vi "LabVIEW-Int_Buck_Boost_Inverter_PI_v0.3.2_9Aug2020.vi"() -> ()   [LabVIEW 2018]
uses:
  <vilib>/Modbus/master/Create Master Instance (TCP).vi
  <vilib>/Modbus/master/Create Master Instance (Serial).vi
  <vilib>/Modbus/master/Modbus Master.lvclass
panel:
  out "Future_5":sgl=1257163500000.0
  out "Future_6":sgl=-2.1506243e+28
  out "Future_4":sgl=84.72166
  out "Future_2":sgl=1.1313919e+38
  out "Future_3":sgl=5.1706567e-10
  out "RMS_V_CA":sgl=1.8692774
  out "Future_1":sgl=3.3164534e-12
  out "RMS_V_BC":sgl=1.8672488
  out "Avg_F_Grid":sgl=60.10614
  out "RMS_V_AB":sgl=1.5779244
  out "Avg_V_Boost":sgl=23.65672
  out "Avg_I_Boost":sgl=-0.037957944
  out "Avg_I_Buck":sgl=0.064867415
  out "Avg_I_DC_In":sgl=0.2081415
  out "Avg_V_Buck":sgl=0.6698118
  out "spll1.theta":sgl=0.025031969
  out "Avg_V_DC_In":sgl=23.77852
  out "Step_sin":sgl=2.9028316
  out "Sine2":sgl=45.3112
  out "Sine3":sgl=1937.8336
  out "V_CA":sgl=0.9757843
  out "Sine1":sgl=1390.5049
  out "V_BC":sgl=-0.4336853
  out "SPI-ADC2_V7":sgl
  out "V_AB":sgl=-0.542099
  out "SPI-ADC2_V5":sgl
  out "SPI-ADC2_V6":sgl
  out "SPI-ADC2_V4":sgl
  out "SPI-ADC2_V2":sgl
  out "SPI-ADC2_V3":sgl
  out "SPI-ADC2_V0":sgl
  out "SPI-ADC2_V1":sgl
  out "SPI-ADC1_V6":sgl
  out "SPI-ADC1_V7":sgl
  out "SPI-ADC1_V5":sgl
  out "SPI-ADC1_V3":sgl
  out "SPI-ADC1_V4":sgl
  out "SPI-ADC1_V1":sgl
  out "SPI-ADC1_V2":sgl
  out "SPI-ADC1_V0":sgl
  out "Ia":sgl=0.07590008
  out "I_L5":sgl=0.009900093
  out "I_Buck":sgl=0.0692997
  out "I_Boost":sgl=-0.0033006668
  out "I_L3":sgl=0.029699326
  out "I_L1":sgl=0.0692997
  out "I_L2":sgl=0.082499504
  out "ADCB7":sgl
  out "I_DCin2":sgl=-0.06270027
  out "ADCB6":sgl
  out "ADCB4":sgl
  out "ADCB5":sgl
  out "ADCB2":sgl
  out "ADCB3":sgl
  out "V_DCin":sgl=23.53728
  out "V_PhA":sgl=-0.7824631
  out "V_PhC":sgl=1.114891
  out "V_PhB":sgl=-1.1619263
  out "V_Buck":sgl=0.64584
  out "I_DCin":sgl=0.23429966
  out "V_Boost":sgl=23.322
  out "ADCB0":sgl
  out "V_Pot":sgl=0.030416729
  out "ADCB1":sgl
  out "Status_Registers":u16[](array[numeric])
  out "DL_RegValues":u16[](array[numeric])=[49325, 30936, 49424, 55648, 49396, 39032, 49437, 56332, 49509, 55732, 49416, 11504, 49415, 20192, 49485, 36984, 49430, 3488, 49418, 50960, 49456, 61696, 49523, 47720, 49458, 44316, 49377, 33664, 49468, 14228, 49465, 40308, 49398, 21648, 49417, 59656, 49479, 32296, 49482, 6216, 49496, 55056, 49468, 14228, 49510, 47040, 49454, 22240, 49490, 50364, 49453, 30928, 49430, 60336, 49430, 60336, 49438, 47632, 49410, 6816, 49440, 30256, 49289, 2800]
  out "Array":sgl[](array[numeric])=[1678.6465, 1616.1086, 1551.6309, 1485.4673, 1417.8794, 1349.1339, 1279.5023, 1209.259, 1138.6813, 1068.048, 997.6377, 927.7282, 858.59503, 790.512, 723.7472, 658.5642, 595.22015, 533.9653, 475.041, 418.67975, 365.1046, 314.5266, 267.1455, 223.14833, 182.70808, 145.98491, 113.12389, 84.2547, 59.490856, 38.93016, 22.654057, 10.726688, 3.1949756, 0.08881263, 1.4203317, 7.184372, 17.358076, 31.901361, 50.756786, 73.85028, 101.09016, 132.36922, 167.56369, 206.53542, 249.12988, 295.1792, 344.50198, 396.90262, 452.1756, 510.1018, 570.45294, 632.99084, 697.4691, 763.6325, 831.2203, 899.96564, 969.59735, 1039.8402, 1110.4181, 1152.81, 1223.3429, 1293.4861, 1362.9624, 1431.4979, 1498.822, 1564.6691, 1628.7792, 1690.8993, 1750.7843, 1808.1979, 1862.9133, 1914.7147, 1963.398, 2008.7705, 2050.6533, 2088.8813, 2123.3037, 2153.7842, 2180.203, 2202.4556, 2220.454, 2234.1277, 2243.422, 2248.3008, 2248.7446, 2244.752, 2236.3381, 2223.5369, 2206.3982, 2184.99, 2159.3965, 2129.7195, 2096.075, 2058.5967, 2017.432, 1972.7434, 1924.7074, 1873.5137, 1819.3641, 1762.4723, 1703.0629, 1641.3706, 1577.6385, 1512.1184, 1445.0685, 1376.7539, 1307.4437, 1237.412, 1166.9349, 1096.2902, 1025.7573, 955.61383, 886.1375, 817.6021, 750.27795, 684.431, 620.32104, 558.2009, 498.31558, 440.90207, 386.18668, 334.38516, 285.70212, 240.32965, 198.44649, 160.21844, 125.79642, 95.31566, 68.89695, 46.64446, 28.645927, 14.972402, 5.6778417, 0.79904556, 0.35511646, 4.3479314, 12.761537, 25.563023, 42.701714, 64.10992, 89.70303, 119.380196, 153.02469, 190.50308, 231.66771, 276.35614, 324.39224, 375.586, 429.73557, 486.62726, 546.0365, 607.7292, 671.4613, 736.9814, 804.0311, 872.3454, 941.6553, 1011.6875, 1082.1652, 1124.5499, 1195.161, 1265.4934, 1335.2695, 1404.2141, 1472.0549, 1538.5243, 1603.3599, 1666.306, 1727.1139, 1785.5438, 1841.365, 1894.3573, 1944.3115, 1991.0305, 2034.3298, 2074.0388, 2110.0005, 2142.0732, 2170.13, 2194.0603, 2213.77, 2229.181, 2240.2324, 2246.8806, 2249.0999, 2246.8809, 2240.2324, 2229.181, 2213.77, 2194.0603, 2170.1301, 2142.0732, 11.81778, 11.655151, 10.083061, 12.576717, 12.79356, 8.782017, 12.847767, 6.722042, 7.80624, 7.8604507, 8.294132, 5.9630966, 3.7947006, 5.7462616, 4.391014, 2.4394493, 1.4636726, -0.10841751, 2.331028, -3.5778618, -2.3852425, -2.7647057, -4.662056, -6.4509926, -5.6378365, -9.595173, -10.896214, -13.552502, -14.203022, -16.8051, -14.745121, -12.305668, -16.20879, -17.835094, -20.166122, -17.78088, -19.73244, -16.371422, -19.461388, -19.190342, -20.708221, -18.485611, -18.756657, -16.371418, -19.407177, -17.997715, -18.75666, -17.83509, -16.15458, -16.58826, -14.257233, -16.750885, -13.606712, -18.106136, -13.823547, -12.522507, -12.739349, -14.203026, -14.148811, -12.305664, -11.709358, -11.329895, -10.733582, -7.6978226, -7.643608, -10.028854, -9.703587, -8.40255, -5.0957413, -6.993088, -5.475212, -5.2583694, -6.234146, -2.276825, -0.2710495, 0.8131485, 2.5478668, 3.6862793, 5.3125763, 6.396782, 10.950417, 8.239922, 9.595169, 8.998863, 13.010403, 11.546734, 13.931969, 10.245693, 14.040386, 10.516739, 15.070381, 11.926201, 10.787788, 11.54673, 10.462528, 11.438309, 9.812008, 13.173031, 13.769337, 11.167263, 8.836227, 9.595173, 12.197254, 9.378334, 12.847771, 11.004627, 9.812012, 11.329891, 8.619392, 8.890438, 8.40255, 7.0472984, 8.998856, 4.824688, 3.4152298, 4.5536423, 4.1741676, 2.8189201, -3.198391, -1.3010406, -0.542099, -2.6020813, -1.409462, -6.55941, -8.023079, -7.752033, -12.739349, -13.877758, -11.81778, -13.44408, -15.449848, -13.498287, -15.93774, -19.35297, -17.45562, -19.08192, -19.136127, -19.298756, -20.057697, -21.955048, -20.437168, -19.786652, -18.377193, -16.750893, -15.612484, -16.859314, -21.467163, -16.750893, -16.47984, -17.40141, -15.124588, -14.8535385, -15.775108, -15.124592, -14.528282, -17.238777, -12.847771, -13.606712, -14.745121, -10.137268, -12.901978, -12.414085, -10.950417, -9.757797, -7.8062363, -13.227238, -8.077293, -6.3425674, -7.914665, -5.6378403, -3.361023, -4.7162704, -3.3610153, -1.8973465, 0.43367767, -0.05420685, -1.1384125, 1.3552475, 4.7704773, 7.8604507, 7.1015167, 9.32412, 10.408325, 8.456757, 13.660919, 11.655148, 13.660923, 12.305668, 14.961956, 11.275677, 14.203022, 12.685139, -15.341431, -13.11882, -13.38987, -16.100368, -14.961964, -15.178799, -15.341427, -17.889301, -15.829319, -15.341431, -19.949284, -17.292992, -17.076149, -18.702446, -16.046158, -16.913525, -15.28722, -15.558273, -18.810871, -13.7693405, -15.016167, -13.11882, -12.4683, -10.625153, -13.498291, -12.847763, -9.486748, -6.396782, -6.5051956, -3.4152298, -4.933113, -3.903122, -0.8131485, -0.7047272, 1.8431473, 2.7647095, 2.276825, 0.8131561, 3.8489075, 5.90889, 6.993088, 9.107285, 8.023079, 7.860443, 9.378326, 10.950417, 14.745125, 11.384102, 14.8535385, 12.305672, 11.438309, 13.823547, 14.582493, 15.666687, 13.931969, 17.13036, 16.696682, 20.870853, 20.057705, 19.895065, 16.85931, 19.895073, 19.786648, 19.515602, 18.322979, 17.618252, 15.504059, 16.15458, 17.50983, 14.36565, 15.829319, 13.552498, 14.203018, 12.847771, 12.576721, 10.679371, 8.890438, 10.841999, 6.938881, 7.0472946, 4.282593, 3.1441803, 1.8431435, 2.2226105, 1.1926193, -1.029995, 0.0, -0.704731, -5.854679, -5.7462616, -8.239922, -8.348343, -7.2099304, -8.782021, -10.841999, -9.757797, -6.5051994, -12.685139, -16.154583, -11.709362, -13.7693405, -11.980412, -11.655148, -14.8535385, -16.317207, -18.214558, -14.8535385, -14.582485, -18.919289, -18.4314, -14.257233, -16.913517, -19.29876, -17.021938, -16.85931, -18.214561, -17.835087, -18.648243, -13.606705, -13.335663, -14.203018, -10.516739, -14.04039, -15.124588, -12.630928, -6.938881, -7.155716, -4.824692, -9.649376, -7.8062363, -1.8431396, -9.757805, -2.7647095, -0.6505203, -2.3852386, -0.8131485, 3.9031143, 3.9031143, 3.7947006, 4.9331055, 8.239914, 8.673599, 8.348343, 5.8004684, 10.950424, 10.354111, 10.462532, 10.137268, 12.739349, 14.257233, 10.950417, 13.7693405, 15.991951, 14.365654, 16.642471, 18.594028, 17.13036, 16.371418, 19.94928, 17.50983, 18.322979, 21.467155, 18.594028, 19.62402, 22.171886, 21.738209, 16.53405, 19.190338, 17.292992, 14.3114395, 14.419861, 19.94928, 14.528278, 8.944649, 11.329891, 11.655148, 8.836235, 7.264145, 7.6978226, 4.7704773, 6.450989, 2.4394493, 4.0115356, 2.4394531, -0.48788834, -0.8131523, -4.228382, -2.873127, -5.0415306, -3.1441765, -4.1741676, -8.402554, 3.5236511, 1.4636688, 3.3068085, 3.5236511, 2.1684036, 6.396782, 2.49366, 11.167259, 8.023079, 7.48098, 11.655151, 11.329895, 13.281448, 12.956184, 11.655144, 14.474075, 13.823547, 15.666691, 16.479843, 17.347202, 17.40141, 15.883526, 17.130356, 17.076145, 19.136127, 22.442936, 20.382961, 19.949284, 20.708218, 20.22033, 19.678234, 16.20879, 17.021938, 18.539822, 18.322975, 15.0161705, 17.455616, 15.558266, 15.61248, 13.281452, 13.715134, 9.378326, 10.733578, 8.510975, 10.028851, 7.0472984, 4.0115356, 6.450989, 1.3010406, 4.282589, 2.818924, 2.9273376, -0.9757805, 2.4394493, -0.108421326, -4.607853, -3.9573326, -6.6678276, -5.9088936, -7.5894012, -5.149952, -8.565178, -9.053066, -11.81778, -10.679371, -7.5893974, -5.8004723, -7.7520294, -12.414089, -7.3725624, -10.354107, -8.294128, -7.968872, -10.570946, -12.305672, -11.492519, -11.438305, -14.528278, -12.251457, -13.444077, -15.233009, -11.384102, -11.438313, -11.221474, -14.203022, -10.516739, -13.931969, -9.540962, -8.185707, -4.7704773, -6.8304596, -3.577858, -3.577858, -2.7647095, 0.37947083, -1.6805115, -3.3068085, -0.48789215, 2.3852463, 0.542099, 4.933113, 2.3852386, -0.5421066, 5.4752045, 3.4694366, 7.2099304, 5.041527, 3.252594, 10.299896, 9.540962, 5.854683, 9.866219, 10.299904, 12.19725, 13.44408, 13.660919, 13.660919, 15.829323, 16.805096, 14.6367035, 14.745117, 13.11882, 15.449852, 21.683998, 20.654007, 14.690914, 19.895065, 18.70245, 21.467155, 21.250317, 17.292988, 23.256092, 18.70245, 20.00349, 19.840858, 19.89507, 15.233013, 15.395641, 16.262997, 17.021942, 12.197254, 11.113052, 10.028851, 10.950424, 4.66206, 6.5052032, 11.004631, 6.6136246, 3.74049, 3.1441765, 4.1741714, 1.084198, -0.21684265, 0.75893784, -2.1141891, -1.3552513, -4.282589, -2.7647057, -5.204159, -7.3725624, -5.4210014, -9.05307, -7.643612, -9.866222, -14.36565, -8.510971, -8.456757, -12.847771, -9.378326, -8.673599, -11.058838, -15.233009, -11.167263, -7.0473022, -11.763569, -11.600941, -7.6978226, -8.619392, -12.4683, -12.630928, -13.5525055, -11.763569, -14.419861, -10.89621, -13.173031, -10.841995, -9.432541, -9.432541, -9.920425, -8.1315, -10.028854, -4.282585]
  out "output array":u16[](array[numeric])=[17617, 54448, 17610, 890, 17601, 62512, 17593, 44788, 17585, 15396, 17576, 42057, 17567, 61459, 17559, 10314, 17550, 21965, 17541, 33161, 17529, 26832, 17511, 61083, 17494, 42517, 17477, 41157, 17460, 61394, 17444, 42012, 17428, 52759, 17413, 32199, 17389, 34111, 17361, 22274, 17334, 36196, 17309, 17256, 17285, 37536, 17247, 9721, 17206, 46405, 17169, 64547, 17122, 16239, 17064, 33384, 17005, 63139, 16923, 47228, 16821, 15234, 16683, 41092, 16460, 31355, 15797, 58213, 16309, 52590, 16613, 58976, 16778, 56663, 16895, 13821, 16971, 1779, 17043, 45912, 17098, 11817, 17156, 24197, 17191, 36942, 17230, 35089, 17273, 8512, 17299, 38640, 17324, 16449, 17350, 29577, 17378, 5754, 17407, 3336, 17422, 40189, 17438, 16234, 17454, 24070, 17470, 59515, 17487, 52761, 17504, 64973, 17522, 26171, 17537, 64227, 17546, 52577, 17552, 6636, 17560, 60153, 17569, 44942, 17578, 24268, 17586, 61423, 17595, 23118, 17603, 38249, 17611, 39151, 17619, 23751, 17626, 55577, 17634, 1621, 17640, 56634, 17647, 22239, 17653, 27836, 17659, 6312, 17664, 10868, 17666, 36378, 17668, 46300, 17670, 40076, 17672, 17215, 17673, 42826, 17674, 51012, 17675, 41483, 17676, 14017, 17676, 34000, 17676, 35818, 17676, 19464, 17675, 50537, 17674, 63639, 17673, 58975, 17672, 36823, 17670, 63064, 17669, 7043, 17667, 307, 17664, 43404, 17660, 11731, 17654, 38858, 17648, 38563, 17642, 12400, 17635, 27559, 17628, 20253, 17620, 57859, 17613, 11228, 17605, 13423, 17597, 970, 17588, 41521, 17580, 6176, 17571, 28211, 17562, 44335, 17553, 56811, 17545, 2377, 17536, 14396, 17518, 59209, 17501, 35021, 17484, 26249, 17467, 37322, 17451, 7062, 17435, 5260, 17419, 36060, 17401, 10341, 17372, 29559, 17345, 6117, 17319, 12621, 17294, 55775, 17264, 21604, 17222, 29261, 17184, 14316, 17147, 38852, 17086, 41374, 17033, 52029, 16954, 37869, 16869, 10972, 16751, 36597, 16565, 45281, 16204, 36416, 16053, 53715, 16523, 8769, 16716, 12097, 16844, 33042, 16938, 52878, 17024, 14407, 17075, 26612, 17134, 49833, 17177, 1618, 17214, 32970, 17255, 43759, 17290, 11670, 17314, 12853, 17339, 51970, 17366, 56871, 17395, 20554, 17416, 33366, 17431, 61099, 17447, 56710, 17464, 16079, 17481, 510, 17498, 5659, 17515, 27120, 17532, 60416, 17543, 17737, 17548, 37273, 17557, 25895, 17566, 12234, 17574, 59552, 17583, 34522, 17592, 450, 17600, 20679, 17608, 27524, 17616, 18891, 17623, 58277, 17631, 12647, 17638, 11182, 17644, 52079, 17651, 2552, 17656, 57594, 17662, 19086, 17665, 41119, 17667, 57346, 17669, 57644, 17671, 41492, 17673, 8439, 17674, 23634, 17675, 21221, 17676, 952, 17676, 28183, 17676, 37273, 17676, 28184, 17676, 952, 17675, 21221, 17674, 23634, 17673, 8439, 17671, 41493, 17669, 57644, 16701, 5536, 16698, 31616, 16673, 21560, 16713, 14908, 16716, 45676, 16652, 33572, 16717, 36980, 16599, 6904, 16633, 52408, 16635, 35024, 16644, 46276, 16574, 53680, 16498, 56416, 16567, 57696, 16524, 33584, 16412, 8176, 16315, 22944, 48606, 2560, 16405, 12176, 49252, 64432, 49176, 42960, 49200, 61680, 49301, 12176, 49358, 28296, 49332, 26920, 49433, 34260, 49454, 22244, 49496, 55052, 49507, 16276, 49542, 28888, 49515, 60420, 49476, 58372, 49537, 43930, 49550, 44614, 49569, 21560, 49550, 16190, 49565, 56330, 49538, 63660, 49563, 45292, 49561, 34258, 49573, 43632, 49555, 57992, 49558, 3490, 49538, 63658, 49563, 16870, 49551, 64338, 49558, 3492, 49550, 44612, 49537, 15508, 49540, 46274, 49508, 7584, 49542, 464, 49497, 46360, 49552, 55646, 49501, 11584, 49480, 23600, 49483, 54368, 49507, 16280, 49506, 24968, 49476, 58368, 49467, 22920, 49461, 18240, 49451, 48320, 49398, 21648, 49396, 39024, 49440, 30256, 49435, 16868, 49414, 28888, 49315, 4176, 49375, 51040, 49327, 13552, 49320, 17552, 49351, 32288, 49169, 46976, 48778, 50944, 16208, 10880, 16419, 4160, 16491, 60416, 16554, 160, 16588, 45680, 16687, 13544, 16643, 54968, 16665, 34256, 16655, 64344, 16720, 10908, 16696, 49004, 16734, 59736, 16675, 61020, 16736, 42348, 16680, 17552, 16753, 8264, 16702, 53688, 16684, 39624, 16696, 49000, 16679, 26244, 16695, 848, 16668, 65020, 16722, 50364, 16732, 20276, 16690, 44316, 16653, 24880, 16665, 34260, 16707, 10228, 16662, 3496, 16717, 36984, 16688, 4852, 16668, 65024, 16693, 18236, 16649, 59656, 16654, 16188, 16646, 28888, 16609, 33656, 16655, 64336, 16538, 25560, 16474, 37664, 16529, 46960, 16517, 37576, 16436, 26928, 49228, 45680, 49062, 34944, 48906, 50944, 49190, 34944, 49076, 26944, 49361, 59056, 49408, 24200, 49400, 4264, 49483, 54368, 49502, 2892, 49469, 5536, 49495, 6900, 49527, 12948, 49495, 63740, 49535, 252, 49562, 53986, 49547, 42268, 49560, 42950, 49561, 5834, 49562, 25562, 49568, 30250, 49583, 41968, 49571, 32594, 49566, 19216, 49555, 1150, 49542, 468, 49529, 52412, 49542, 57312, 49579, 48320, 49542, 468, 49539, 54966, 49547, 13846, 49521, 65104, 49517, 43032, 49532, 26328, 49521, 65108, 49512, 29656, 49545, 59652, 49485, 36984, 49497, 46360, 49515, 60420, 49442, 12864, 49486, 28288, 49478, 40984, 49455, 13544, 49436, 8176, 49401, 52400, 49491, 41668, 49409, 15512, 49354, 63056, 49405, 17648, 49332, 26928, 49239, 6912, 49302, 60336, 49239, 6880, 49138, 56384, 16094, 2816, 48478, 2048, 49041, 46976, 16301, 30912, 16536, 42944, 16635, 35024, 16611, 16288, 16661, 12184, 16678, 34944, 16647, 20192, 16730, 37664, 16698, 31612, 16730, 37668, 16708, 58372, 16751, 25644, 16692, 26924, 16739, 16276, 16714, 63060, 49525, 30336, 49489, 59056, 49494, 15592, 49536, 52622, 49519, 25652, 49522, 56412, 49525, 30332, 49551, 7498, 49533, 17636, 49525, 30336, 49567, 38946, 49546, 22540, 49544, 39924, 49557, 40604, 49536, 24200, 49543, 20198, 49524, 39028, 49528, 61104, 49558, 31914, 49500, 20280, 49520, 16952, 49489, 59056, 49479, 32296, 49450, 160, 49495, 63744, 49485, 36976, 49431, 51640, 49356, 45680, 49360, 10896, 49242, 37664, 49309, 56336, 49273, 52416, 48976, 10880, 48948, 26880, 16363, 60480, 16432, 61696, 16401, 46976, 16208, 11008, 16502, 21632, 16573, 5536, 16607, 51040, 16657, 46960, 16640, 24200, 16635, 35008, 16662, 3488, 16687, 13544, 16747, 60424, 16694, 9544, 16749, 43032, 16708, 58376, 16695, 848, 16733, 11584, 16745, 20964, 16762, 43712, 16734, 59736, 16777, 2810, 16773, 37582, 16806, 63362, 16800, 30254, 16799, 10520, 16774, 57310, 16799, 10524, 16798, 19214, 16796, 8180, 16786, 38262, 16780, 61998, 16760, 4256, 16769, 15508, 16780, 5154, 16741, 55732, 16765, 17636, 16728, 55048, 16739, 16272, 16717, 36984, 16713, 14912, 16682, 57012, 16654, 16188, 16685, 30932, 16606, 2896, 16609, 33648, 16521, 2816, 16457, 14912, 16363, 60448, 16398, 16192, 16280, 42944, 49027, 55008, 0, 0, 48948, 26944, 49339, 22920, 49335, 57696, 49411, 54968, 49413, 37584, 49382, 47040, 49420, 33576, 49453, 30932, 49436, 8176, 49360, 10904, 49482, 63060, 49537, 15510, 49467, 22924, 49500, 20280, 49471, 44996, 49466, 31612, 49517, 43032, 49538, 35236, 49553, 46954, 49517, 43032, 49513, 20956, 49559, 23220, 49555, 29570, 49508, 7584, 49543, 20194, 49562, 25564, 49544, 11502, 49542, 57310, 49553, 46956, 49550, 44610, 49557, 12186, 49497, 46352, 49493, 24288, 49507, 16272, 49448, 17552, 49504, 42352, 49521, 65104, 49482, 6216, 49374, 2896, 49380, 64416, 49306, 25568, 49434, 25560, 49401, 52400, 49131, 60416, 49436, 8184, 49200, 61696, 48934, 34944, 49176, 42944, 48976, 10880, 16505, 52384, 16505, 52384, 16498, 56416, 16541, 56320, 16643, 54960, 16650, 50960, 16645, 37584, 16569, 40304, 16687, 13552, 16677, 43632, 16679, 26248, 16674, 12864, 16715, 54368, 16740, 7584, 16687, 13544, 16732, 20280, 16767, 57096, 16741, 55736, 16773, 9160, 16788, 49298, 16777, 2810, 16770, 63658, 16799, 38944, 16780, 5154, 16786, 38262, 16811, 48316, 16788, 49298, 16796, 65022, 16817, 24582, 16813, 59354, 16772, 17852, 16793, 34256, 16778, 22540, 16740, 64424, 16742, 47040, 16799, 38944, 16744, 29652, 16655, 7496, 16693, 18236, 16698, 31612, 16653, 24888, 16616, 29664, 16630, 21648, 16536, 42944, 16590, 28288, 16412, 8176, 16512, 24192, 16412, 8192, 48889, 52352, 48976, 10944, 49287, 20200, 49207, 57680, 49313, 21560, 49225, 14896, 49285, 37576, 49414, 28892, 16481, 33664, 16315, 22912, 16467, 41664, 16481, 33664, 16394, 50976, 16588, 45680, 16415, 38944, 16690, 44312, 16640, 24200, 16623, 25648, 16698, 31616, 16693, 18240, 16724, 32976, 16719, 19592, 16698, 31608, 16743, 38352, 16733, 11584, 16762, 43716, 16771, 54968, 16778, 50962, 16779, 13846, 16766, 8940, 16777, 2808, 16776, 39922, 16793, 5834, 16819, 35618, 16803, 4174, 16799, 38946, 16805, 43630, 16801, 49980, 16797, 27910, 16769, 43930, 16776, 11502, 16788, 20878, 16786, 38260, 16752, 16956, 16779, 42266, 16760, 61096, 16761, 52408, 16724, 32980, 16731, 28976, 16662, 3488, 16683, 48316, 16648, 11508, 16672, 30252, 16609, 33656, 16512, 24192, 16590, 28288, 16294, 34944, 16521, 2808, 16436, 26944, 16443, 22912, 49017, 52416, 16412, 8176, 48606, 3072, 49299, 29576, 49277, 17648, 49365, 24280, 49341, 5544, 49394, 56416, 49316, 52328, 49417, 2808, 49424, 55644, 49469, 5536, 49450, 57012, 49394, 56408, 49337, 40312, 49400, 4256, 49478, 40988, 49387, 60424, 49445, 43628, 49412, 46272, 49407, 256, 49449, 8856, 49476, 58376, 49463, 57692, 49463, 844, 49512, 29652, 49476, 1528, 49495, 6896, 49523, 47720, 49462, 9544, 49463, 852, 49459, 35624, 49507, 16276, 49448, 17552, 49502, 59736, 49432, 42952, 49410, 63656, 49304, 42944, 49370, 37664, 49252, 64416, 49252, 64416, 49200, 61696, 16066, 18944, 49111, 6912, 49235, 41664, 48889, 52480, 16408, 42976, 16138, 50944, 16541, 56336, 16408, 42944, 48906, 51072, 16559, 13536, 16478, 2880, 16614, 47040, 16545, 21552, 16464, 10880, 16676, 52320, 16664, 42952, 16571, 22928, 16669, 56328, 16676, 52328, 16707, 10224, 16727, 6900, 16730, 37664, 16730, 37664, 16765, 17640, 16774, 28886, 16746, 12272, 16747, 60416, 16721, 59056, 16759, 12952, 16813, 30932, 16805, 15208, 16747, 3580, 16799, 10520, 16789, 40606, 16811, 48316, 16810, 166, 16778, 22538, 16826, 3194, 16789, 40606, 16800, 1830, 16798, 47636, 16799, 10522, 16755, 47724, 16758, 21644, 16770, 6814, 16776, 11504, 16707, 10228, 16689, 53008, 16672, 30252, 16687, 13552, 16533, 12184, 16592, 10912, 16688, 4856, 16595, 41680, 16495, 25648, 16457, 14896, 16517, 37584, 16266, 50944, 48734, 3072, 16194, 18880, 49159, 20192, 49069, 30944, 49289, 2808, 49200, 61680, 49318, 34936, 49387, 60424, 49325, 30936, 49424, 55648, 49396, 39032, 49437, 56332, 49509, 55732, 49416, 11504, 49415, 20192, 49485, 36984, 49430, 3488, 49418, 50960, 49456, 61696, 49523, 47720, 49458, 44316, 49377, 33664, 49468, 14228, 49465, 40308, 49398, 21648, 49417, 59656, 49479, 32296, 49482, 6216, 49496, 55056, 49468, 14228, 49510, 47040, 49454, 22240, 49490, 50364, 49453, 30928, 49430, 60336, 49430, 60336, 49438, 47632, 49410, 6816, 49440, 30256, 49289, 2800]
  in  "ARA-SGPN Interface Demo":enum32{"Control", "Datalogger"}(tab)
  in  "parity (None)":u16(ring) items=["None", "Odd", "Even"]
  in  "baud rate (115200)":u32=115200
  in  "unit ID":u8=1
  in  "serial type":enum16{"RTU", "ASCII"}(ring)
  in  "Serail Comm Port":refnum<visa-resource-name>="COM13"
  out "RX/TX_Errors":i16=52
  out "Modbus_Master-Error":errorcluster
  in  "IP Address":string="192.168.0.64"
  in  "CtrlSrc_Serial/nTCP":bool=TRUE
  in  "Inverter_Op-Mode":u16(ring)=1 items=["Passive", "Islanded", "Grid-Forming", "Grid-Feeding", "Grid-Supporting"]
  in  "AC Mag Ref (V)":fxp<+,16,11>=30.0
  in  "PWM_En":bool
  in  "PLL_Ki":fxp<+,16,6>=0.009765625
  in  "AC Power Ref (Q)":fxp<+,16,6>
  in  "PLL_Kp":fxp<+,16,6>=1.0
  in  "AC Freq Ref (Hz)":fxp<+,16,11>=60.0
  in  "AC Power Ref (P)":fxp<+,16,6>
  in  "Inv_Sw_Freq (kHz)":fxp<+,16,11>=30.0
  in  "Inv_En":bool
  in  "Buck_En":bool
  in  "Boost_En":bool
  in  "Buck_Op-Mode":u16(ring)=1 items=["Passive", "Voltage-Mode", "Current-Mode", "Dual-Loop"]
  in  "Buck_V_Ref (V)":fxp<+,16,6>=15.0
  in  "Buck_I_Kp":fxp<+,16,6>=1.0
  in  "Buck_V_Ki":fxp<+,16,6>=0.03125
  in  "Buck_I_Ki":fxp<+,16,6>=0.009765625
  in  "Buck_I_Ref (A)":fxp<+,16,6>
  in  "Buck_V_Kp":fxp<+,16,6>=1.0
  in  "Buck_Sw_Freq (kHz)":fxp<+,16,11>=30.0
  in  "Boost_Op-Mode":u16(ring)=1 items=["Passive", "Voltage-Mode", "Current-Mode", "Dual-Loop"]
  in  "Boost_V_Ref (V)":fxp<+,16,6>=36.0
  in  "Boost_I_Ki":fxp<+,16,6>=0.009765625
  in  "Boost_V_Ki":fxp<+,16,6>=0.03125
  in  "Boost_I_Ref (A)":fxp<+,16,6>
  in  "Boost_V_Kp":fxp<+,16,6>=1.0
  in  "Boost_Sw_Freq (kHz)":fxp<+,16,11>=30.0
  in  "Boost_I_Kp":fxp<+,16,6>=1.0
  out "V_Buck_FP":sgl=0.64584
  out "V_Boost_FP":sgl=23.322
  out "I_Boost_FP":sgl=-0.0033006668
  out "I_Buck_FP":sgl=0.0692997
  out "V_DCin_FP":sgl=23.53728
  out "I_DCin_FP":sgl=0.23429966
  out "V_Pot_FP":sgl=0.030416729
  out "RMS_V_AB_FP":sgl=1.5779244
  out "Avg_F_Grid_FP":sgl=60.10614
  out "RMS_V_BC_FP":sgl=1.8672488
  out "RMS_V_CA_FP":sgl=1.8692774
  in  "Chan_4":u16(ring)=42 items=["V_DCin", "V_PhA", "V_PhB", "V_PhC", "V_Buck", "V_Boost", "I_DCin", "V_Pot", "ADCB0", "ADCB1", "ADCB2", "ADCB3", "ADCB4", "ADCB5", "ADCB6", "ADCB7", "I_DCin2", "I_L1", "I_L2", "I_L3", "I_Buck", "I_Boost", "Ia", "I_L5", "SPI-ADC1_V0", "SPI-ADC1_V1", "SPI-ADC1_V2", "SPI-ADC1_V3", "SPI-ADC1_V4", "SPI-ADC1_V5", "SPI-ADC1_V6", "SPI-ADC1_V7", "SPI-ADC2_V0", "SPI-ADC2_V1", "SPI-ADC2_V2", "SPI-ADC2_V3", "SPI-ADC2_V4", "SPI-ADC2_V5", "SPI-ADC2_V6", "SPI-ADC2_V7", "V_AB", "V_BC", "V_CA", "Sine1", "Sine2", "Sine3", "Step_sin", "spll1.theta", "Avg_V_DC_In", "Avg_I_DC_In", "Avg_V_Buck", "Avg_I_Buck", "Avg_V_Boost", "Avg_I_Boost", "Avg_F_Grid", "RMS_V_AB", "RMS_V_BC", "RMS_V_CA"]
  in  "Chan_3":u16(ring)=41 items=["V_DCin", "V_PhA", "V_PhB", "V_PhC", "V_Buck", "V_Boost", "I_DCin", "V_Pot", "ADCB0", "ADCB1", "ADCB2", "ADCB3", "ADCB4", "ADCB5", "ADCB6", "ADCB7", "I_DCin2", "I_L1", "I_L2", "I_L3", "I_Buck", "I_Boost", "Ia", "I_L5", "SPI-ADC1_V0", "SPI-ADC1_V1", "SPI-ADC1_V2", "SPI-ADC1_V3", "SPI-ADC1_V4", "SPI-ADC1_V5", "SPI-ADC1_V6", "SPI-ADC1_V7", "SPI-ADC2_V0", "SPI-ADC2_V1", "SPI-ADC2_V2", "SPI-ADC2_V3", "SPI-ADC2_V4", "SPI-ADC2_V5", "SPI-ADC2_V6", "SPI-ADC2_V7", "V_AB", "V_BC", "V_CA", "Sine1", "Sine2", "Sine3", "Step_sin", "spll1.theta", "Avg_V_DC_In", "Avg_I_DC_In", "Avg_V_Buck", "Avg_I_Buck", "Avg_V_Boost", "Avg_I_Boost", "Avg_F_Grid", "RMS_V_AB", "RMS_V_BC", "RMS_V_CA"]
  in  "Chan_2":u16(ring)=40 items=["V_DCin", "V_PhA", "V_PhB", "V_PhC", "V_Buck", "V_Boost", "I_DCin", "V_Pot", "ADCB0", "ADCB1", "ADCB2", "ADCB3", "ADCB4", "ADCB5", "ADCB6", "ADCB7", "I_DCin2", "I_L1", "I_L2", "I_L3", "I_Buck", "I_Boost", "Ia", "I_L5", "SPI-ADC1_V0", "SPI-ADC1_V1", "SPI-ADC1_V2", "SPI-ADC1_V3", "SPI-ADC1_V4", "SPI-ADC1_V5", "SPI-ADC1_V6", "SPI-ADC1_V7", "SPI-ADC2_V0", "SPI-ADC2_V1", "SPI-ADC2_V2", "SPI-ADC2_V3", "SPI-ADC2_V4", "SPI-ADC2_V5", "SPI-ADC2_V6", "SPI-ADC2_V7", "V_AB", "V_BC", "V_CA", "Sine1", "Sine2", "Sine3", "Step_sin", "spll1.theta", "Avg_V_DC_In", "Avg_I_DC_In", "Avg_V_Buck", "Avg_I_Buck", "Avg_V_Boost", "Avg_I_Boost", "Avg_F_Grid", "RMS_V_AB", "RMS_V_BC", "RMS_V_CA"]
  out "DL_Logging":bool
  out "DL_Trig_Wait":bool
  out "DL_Ready":bool=TRUE
  in  "DL_Start":bool
  in  "Chan_1 (Trig)":u16(ring)=43 items=["V_DCin", "V_PhA", "V_PhB", "V_PhC", "V_Buck", "V_Boost", "I_DCin", "V_Pot", "ADCB0", "ADCB1", "ADCB2", "ADCB3", "ADCB4", "ADCB5", "ADCB6", "ADCB7", "I_DCin2", "I_L1", "I_L2", "I_L3", "I_Buck", "I_Boost", "Ia", "I_L5", "SPI-ADC1_V0", "SPI-ADC1_V1", "SPI-ADC1_V2", "SPI-ADC1_V3", "SPI-ADC1_V4", "SPI-ADC1_V5", "SPI-ADC1_V6", "SPI-ADC1_V7", "SPI-ADC2_V0", "SPI-ADC2_V1", "SPI-ADC2_V2", "SPI-ADC2_V3", "SPI-ADC2_V4", "SPI-ADC2_V5", "SPI-ADC2_V6", "SPI-ADC2_V7", "V_AB", "V_BC", "V_CA", "Sine1", "Sine2", "Sine3", "Step_sin", "spll1.theta", "Avg_V_DC_In", "Avg_I_DC_In", "Avg_V_Buck", "Avg_I_Buck", "Avg_V_Boost", "Avg_I_Boost", "Avg_F_Grid", "RMS_V_AB", "RMS_V_BC", "RMS_V_CA"]
  in  "Trig-Level":sgl=1000.0
  in  "Prescaler (Skip)":u16=5
  out "Waveform Graph":dynamicdata(graph)=[{"t0"=timestamp(0 s since 1904-01-01), "dt"=1.0, "Y"=[1678.646484375, 1616.108642578125, 1551.630859375, 1485.46728515625, 1417.87939453125, 1349.1339111328125, 1279.5023193359375, 1209.259033203125, 1138.6812744140625, 1068.0479736328125, 997.6376953125, 927.7282104492188, 858.5950317382812, 790.5120239257812, 723.7471923828125, 658.564208984375, 595.2201538085938, 533.9652709960938, 475.0409851074219, 418.67974853515625, 365.1046142578125, 314.526611328125, 267.1455078125, 223.14833068847656, 182.7080841064453, 145.9849090576172, 113.12389373779297, 84.25469970703125, 59.4908561706543, 38.93016052246094, 22.654056549072266, 10.726688385009766, 3.1949756145477295, 0.08881262689828873, 1.4203317165374756, 7.1843719482421875, 17.358076095581055, 31.9013614654541, 50.75678634643555, 73.85028076171875, 101.09015655517578, 132.3692169189453, 167.56369018554688, 206.53541564941406, 249.1298828125, 295.17919921875, 344.5019836425781, 396.9026184082031, 452.17559814453125, 510.101806640625, 570.4529418945312, 632.9908447265625, 697.4691162109375, 763.6325073242188, 831.2202758789062, 899.9656372070312, 969.5973510742188, 1039.8402099609375, 1110.4180908203125, 1152.81005859375, 1223.3428955078125, 1293.486083984375, 1362.96240234375, 1431.4979248046875, 1498.822021484375, 1564.6690673828125, 1628.7791748046875, 1690.8992919921875, 1750.7843017578125, 1808.1978759765625, 1862.913330078125, 1914.7147216796875, 1963.39794921875, 2008.7705078125, 2050.6533203125, 2088.88134765625, 2123.3037109375, 2153.7841796875, 2180.202880859375, 2202.45556640625, 2220.4541015625, 2234.127685546875, 2243.422119140625, 2248.30078125, 2248.74462890625, 2244.751953125, 2236.338134765625, 2223.536865234375, 2206.398193359375, 2184.989990234375, 2159.396484375, 2129.719482421875, 2096.074951171875, 2058.5966796875, 2017.4320068359375, 1972.743408203125, 1924.7073974609375, 1873.513671875, 1819.3641357421875, 1762.4722900390625, 1703.0628662109375, 1641.37060546875, 1577.6385498046875, 1512.118408203125, 1445.0684814453125, 1376.75390625, 1307.4437255859375, 1237.4119873046875, 1166.9349365234375, 1096.2901611328125, 1025.75732421875, 955.6138305664062, 886.1375122070312, 817.6021118164062, 750.2779541015625, 684.4310302734375, 620.321044921875, 558.200927734375, 498.3155822753906, 440.9020690917969, 386.1866760253906, 334.3851623535156, 285.7021179199219, 240.32965087890625, 198.4464874267578, 160.21844482421875, 125.79641723632812, 95.31565856933594, 68.8969497680664, 46.64445877075195, 28.64592742919922, 14.97240161895752, 5.677841663360596, 0.7990455627441406, 0.35511645674705505, 4.347931385040283, 12.761536598205566, 25.56302261352539, 42.70171356201172, 64.10991668701172, 89.70303344726562, 119.38019561767578, 153.02468872070312, 190.50308227539062, 231.66770935058594, 276.35614013671875, 324.3922424316406, 375.58599853515625, 429.7355651855469, 486.62725830078125, 546.0364990234375, 607.7291870117188, 671.4613037109375, 736.9813842773438, 804.0311279296875, 872.3453979492188, 941.6552734375, 1011.6875, 1082.1651611328125, 1124.5499267578125, 1195.1610107421875, 1265.493408203125, 1335.26953125, 1404.214111328125, 1472.054931640625, 1538.5242919921875, 1603.35986328125, 1666.3060302734375, 1727.1138916015625, 1785.5438232421875, 1841.364990234375, 1894.3572998046875, 1944.3115234375, 1991.030517578125, 2034.329833984375, 2074.038818359375, 2110.00048828125, 2142.0732421875, 2170.1298828125, 2194.060302734375, 2213.77001953125, 2229.180908203125, 2240.232421875, 2246.880615234375, 2249.099853515625, 2246.880859375, 2240.232421875, 2229.180908203125, 2213.77001953125, 2194.060302734375, 2170.130126953125, 2142.0732421875]}, {"t0"=timestamp(0 s since 1904-01-01), "dt"=1.0, "Y"=[11.817779541015625, 11.6551513671875, 10.083061218261719, 12.576717376708984, 12.793560028076172, 8.78201675415039, 12.847766876220703, 6.722042083740234, 7.806240081787109, 7.860450744628906, 8.294132232666016, 5.963096618652344, 3.7947006225585938, 5.7462615966796875, 4.391014099121094, 2.4394493103027344, 1.4636726379394531, -0.10841751098632812, 2.3310279846191406, -3.577861785888672, -2.385242462158203, -2.7647056579589844, -4.662055969238281, -6.450992584228516, -5.637836456298828, -9.595172882080078, -10.89621353149414, -13.552501678466797, -14.203022003173828, -16.805099487304688, -14.745121002197266, -12.305667877197266, -16.208789825439453, -17.835094451904297, -20.166122436523438, -17.780879974365234, -19.732440948486328, -16.371421813964844, -19.461387634277344, -19.19034194946289, -20.708221435546875, -18.485610961914062, -18.756656646728516, -16.371417999267578, -19.407176971435547, -17.99771499633789, -18.75666046142578, -17.83509063720703, -16.154579162597656, -16.588260650634766, -14.257232666015625, -16.750885009765625, -13.606712341308594, -18.106136322021484, -13.82354736328125, -12.522506713867188, -12.739349365234375, -14.203025817871094, -14.148811340332031, -12.3056640625, -11.709358215332031, -11.32989501953125, -10.73358154296875, -7.697822570800781, -7.643608093261719, -10.028854370117188, -9.70358657836914, -8.402549743652344, -5.095741271972656, -6.9930877685546875, -5.475212097167969, -5.258369445800781, -6.2341461181640625, -2.276824951171875, -0.27104949951171875, 0.8131484985351562, 2.5478668212890625, 3.686279296875, 5.3125762939453125, 6.396781921386719, 10.950416564941406, 8.239921569824219, 9.595169067382812, 8.998863220214844, 13.01040267944336, 11.546733856201172, 13.931968688964844, 10.24569320678711, 14.040386199951172, 10.516738891601562, 15.070381164550781, 11.926200866699219, 10.787788391113281, 11.546730041503906, 10.462528228759766, 11.438308715820312, 9.812007904052734, 13.173030853271484, 13.769336700439453, 11.16726303100586, 8.836227416992188, 9.595172882080078, 12.197254180908203, 9.378334045410156, 12.847770690917969, 11.004627227783203, 9.81201171875, 11.329891204833984, 8.619392395019531, 8.890438079833984, 8.402549743652344, 7.047298431396484, 8.998855590820312, 4.824687957763672, 3.4152297973632812, 4.553642272949219, 4.174167633056641, 2.818920135498047, -3.1983909606933594, -1.3010406494140625, -0.5420989990234375, -2.602081298828125, -1.4094619750976562, -6.559410095214844, -8.023078918457031, -7.752033233642578, -12.739349365234375, -13.877758026123047, -11.817779541015625, -13.444080352783203, -15.449848175048828, -13.498287200927734, -15.937740325927734, -19.352970123291016, -17.45561981201172, -19.081920623779297, -19.136127471923828, -19.298755645751953, -20.057697296142578, -21.955047607421875, -20.43716812133789, -19.786651611328125, -18.377193450927734, -16.750892639160156, -15.612483978271484, -16.85931396484375, -21.4671630859375, -16.750892639160156, -16.479839324951172, -17.401409149169922, -15.124588012695312, -14.853538513183594, -15.775108337402344, -15.124591827392578, -14.528282165527344, -17.23877716064453, -12.847770690917969, -13.606712341308594, -14.745121002197266, -10.13726806640625, -12.9019775390625, -12.414085388183594, -10.950416564941406, -9.757797241210938, -7.806236267089844, -13.227237701416016, -8.077293395996094, -6.342567443847656, -7.914665222167969, -5.637840270996094, -3.36102294921875, -4.716270446777344, -3.3610153198242188, -1.8973464965820312, 0.43367767333984375, -0.05420684814453125, -1.1384124755859375, 1.3552474975585938, 4.770477294921875, 7.860450744628906, 7.1015167236328125, 9.324119567871094, 10.4083251953125, 8.456756591796875, 13.660919189453125, 11.655147552490234, 13.66092300415039, 12.305667877197266, 14.961956024169922, 11.275676727294922, 14.203022003173828, 12.685138702392578]}, {"t0"=timestamp(0 s since 1904-01-01), "dt"=1.0, "Y"=[-15.3414306640625, -13.118820190429688, -13.389869689941406, -16.10036849975586, -14.961963653564453, -15.17879867553711, -15.341426849365234, -17.889301300048828, -15.82931900024414, -15.3414306640625, -19.949283599853516, -17.292991638183594, -17.076148986816406, -18.70244598388672, -16.046157836914062, -16.913524627685547, -15.287220001220703, -15.558273315429688, -18.810871124267578, -13.769340515136719, -15.016166687011719, -13.118820190429688, -12.468299865722656, -10.625152587890625, -13.498291015625, -12.847763061523438, -9.486747741699219, -6.396781921386719, -6.505195617675781, -3.4152297973632812, -4.933113098144531, -3.9031219482421875, -0.8131484985351562, -0.7047271728515625, 1.8431472778320312, 2.76470947265625, 2.276824951171875, 0.8131561279296875, 3.848907470703125, 5.9088897705078125, 6.9930877685546875, 9.107284545898438, 8.023078918457031, 7.860443115234375, 9.378326416015625, 10.950416564941406, 14.745124816894531, 11.384101867675781, 14.853538513183594, 12.305671691894531, 11.438308715820312, 13.82354736328125, 14.58249282836914, 15.66668701171875, 13.931968688964844, 17.130359649658203, 16.69668197631836, 20.870853424072266, 20.05770492553711, 19.895065307617188, 16.859310150146484, 19.89507293701172, 19.78664779663086, 19.515602111816406, 18.322978973388672, 17.61825180053711, 15.504058837890625, 16.154579162597656, 17.509830474853516, 14.365650177001953, 15.82931900024414, 13.552497863769531, 14.203018188476562, 12.847770690917969, 12.57672119140625, 10.679370880126953, 8.890438079833984, 10.841999053955078, 6.938880920410156, 7.047294616699219, 4.2825927734375, 3.1441802978515625, 1.8431434631347656, 2.2226104736328125, 1.1926193237304688, -1.0299949645996094, 0.0, -0.7047309875488281, -5.854679107666016, -5.7462615966796875, -8.239921569824219, -8.348342895507812, -7.209930419921875, -8.782020568847656, -10.841999053955078, -9.757797241210938, -6.505199432373047, -12.685138702392578, -16.154582977294922, -11.709362030029297, -13.769340515136719, -11.980411529541016, -11.655147552490234, -14.853538513183594, -16.31720733642578, -18.214557647705078, -14.853538513183594, -14.58248519897461, -18.919288635253906, -18.431400299072266, -14.257232666015625, -16.913516998291016, -19.29875946044922, -17.02193832397461, -16.859310150146484, -18.214561462402344, -17.835086822509766, -18.648242950439453, -13.606704711914062, -13.335662841796875, -14.203018188476562, -10.516738891601562, -14.040390014648438, -15.124588012695312, -12.630928039550781, -6.938880920410156, -7.1557159423828125, -4.8246917724609375, -9.649375915527344, -7.806236267089844, -1.8431396484375, -9.757804870605469, -2.76470947265625, -0.6505203247070312, -2.3852386474609375, -0.8131484985351562, 3.9031143188476562, 3.9031143188476562, 3.7947006225585938, 4.93310546875, 8.239913940429688, 8.673599243164062, 8.348342895507812, 5.800468444824219, 10.950424194335938, 10.354110717773438, 10.462532043457031, 10.13726806640625, 12.739349365234375, 14.257232666015625, 10.950416564941406, 13.769340515136719, 15.991950988769531, 14.365653991699219, 16.642471313476562, 18.59402847290039, 17.130359649658203, 16.371417999267578, 19.94927978515625, 17.509830474853516, 18.322978973388672, 21.46715545654297, 18.59402847290039, 19.624019622802734, 22.171886444091797, 21.738208770751953, 16.53404998779297, 19.190338134765625, 17.292991638183594, 14.311439514160156, 14.41986083984375, 19.94927978515625, 14.528278350830078, 8.944648742675781, 11.329891204833984, 11.655147552490234, 8.836235046386719, 7.2641448974609375, 7.697822570800781, 4.770477294921875, 6.45098876953125, 2.4394493103027344, 4.01153564453125, 2.439453125, -0.4878883361816406, -0.8131523132324219, -4.228382110595703, -2.873126983642578, -5.041530609130859, -3.144176483154297, -4.174167633056641, -8.40255355834961]}, {"t0"=timestamp(0 s since 1904-01-01), "dt"=1.0, "Y"=[3.523651123046875, 1.4636688232421875, 3.3068084716796875, 3.523651123046875, 2.1684036254882812, 6.396781921386719, 2.4936599731445312, 11.167259216308594, 8.023078918457031, 7.480979919433594, 11.6551513671875, 11.32989501953125, 13.281448364257812, 12.956184387207031, 11.655143737792969, 14.474075317382812, 13.82354736328125, 15.666690826416016, 16.479843139648438, 17.34720230102539, 17.401409149169922, 15.883525848388672, 17.130355834960938, 17.07614517211914, 19.136127471923828, 22.442935943603516, 20.38296127319336, 19.949283599853516, 20.70821762084961, 20.22032928466797, 19.678234100341797, 16.208789825439453, 17.02193832397461, 18.53982162475586, 18.322975158691406, 15.016170501708984, 17.455615997314453, 15.558265686035156, 15.612480163574219, 13.281452178955078, 13.715133666992188, 9.378326416015625, 10.733577728271484, 8.510974884033203, 10.028850555419922, 7.047298431396484, 4.01153564453125, 6.45098876953125, 1.3010406494140625, 4.282588958740234, 2.8189239501953125, 2.927337646484375, -0.9757804870605469, 2.4394493103027344, -0.10842132568359375, -4.607852935791016, -3.9573326110839844, -6.667827606201172, -5.908893585205078, -7.5894012451171875, -5.149951934814453, -8.565177917480469, -9.05306625366211, -11.817779541015625, -10.679370880126953, -7.589397430419922, -5.800472259521484, -7.7520294189453125, -12.41408920288086, -7.372562408447266, -10.354106903076172, -8.29412841796875, -7.9688720703125, -10.570945739746094, -12.305671691894531, -11.49251937866211, -11.438304901123047, -14.528278350830078, -12.251457214355469, -13.444076538085938, -15.233009338378906, -11.384101867675781, -11.438312530517578, -11.221473693847656, -14.203022003173828, -10.516738891601562, -13.931968688964844, -9.540962219238281, -8.185707092285156, -4.770477294921875, -6.8304595947265625, -3.5778579711914062, -3.5778579711914062, -2.76470947265625, 0.3794708251953125, -1.680511474609375, -3.3068084716796875, -0.48789215087890625, 2.3852462768554688, 0.5420989990234375, 4.933113098144531, 2.3852386474609375, -0.5421066284179688, 5.4752044677734375, 3.4694366455078125, 7.209930419921875, 5.041526794433594, 3.252593994140625, 10.299896240234375, 9.540962219238281, 5.854682922363281, 9.866218566894531, 10.299903869628906, 12.197250366210938, 13.444080352783203, 13.660919189453125, 13.660919189453125, 15.829322814941406, 16.805095672607422, 14.636703491210938, 14.7451171875, 13.118820190429688, 15.449851989746094, 21.683998107910156, 20.654006958007812, 14.690914154052734, 19.895065307617188, 18.702449798583984, 21.46715545654297, 21.250316619873047, 17.292987823486328, 23.256092071533203, 18.702449798583984, 20.003490447998047, 19.840858459472656, 19.895069122314453, 15.233013153076172, 15.395641326904297, 16.262996673583984, 17.021942138671875, 12.197254180908203, 11.113052368164062, 10.028850555419922, 10.950424194335938, 4.662059783935547, 6.5052032470703125, 11.004631042480469, 6.613624572753906, 3.740489959716797, 3.144176483154297, 4.174171447753906, 1.084197998046875, -0.2168426513671875, 0.7589378356933594, -2.1141891479492188, -1.3552513122558594, -4.282588958740234, -2.7647056579589844, -5.204158782958984, -7.372562408447266, -5.421001434326172, -9.053070068359375, -7.643611907958984, -9.866222381591797, -14.365650177001953, -8.510971069335938, -8.456756591796875, -12.847770690917969, -9.378326416015625, -8.673599243164062, -11.058837890625, -15.233009338378906, -11.16726303100586, -7.04730224609375, -11.763568878173828, -11.600940704345703, -7.697822570800781, -8.619392395019531, -12.468299865722656, -12.630928039550781, -13.552505493164062, -11.763568878173828, -14.41986083984375, -10.896209716796875, -13.173030853271484, -10.841995239257812, -9.432540893554688, -9.432540893554688, -9.920425415039062, -8.131500244140625, -10.028854370117188, -4.282585144042969]}]
  out "DL_Iterations":i32=5
  out "DL_Status":u16
  in  "Trig_Bypass":bool
  in  "Master_Stop":bool
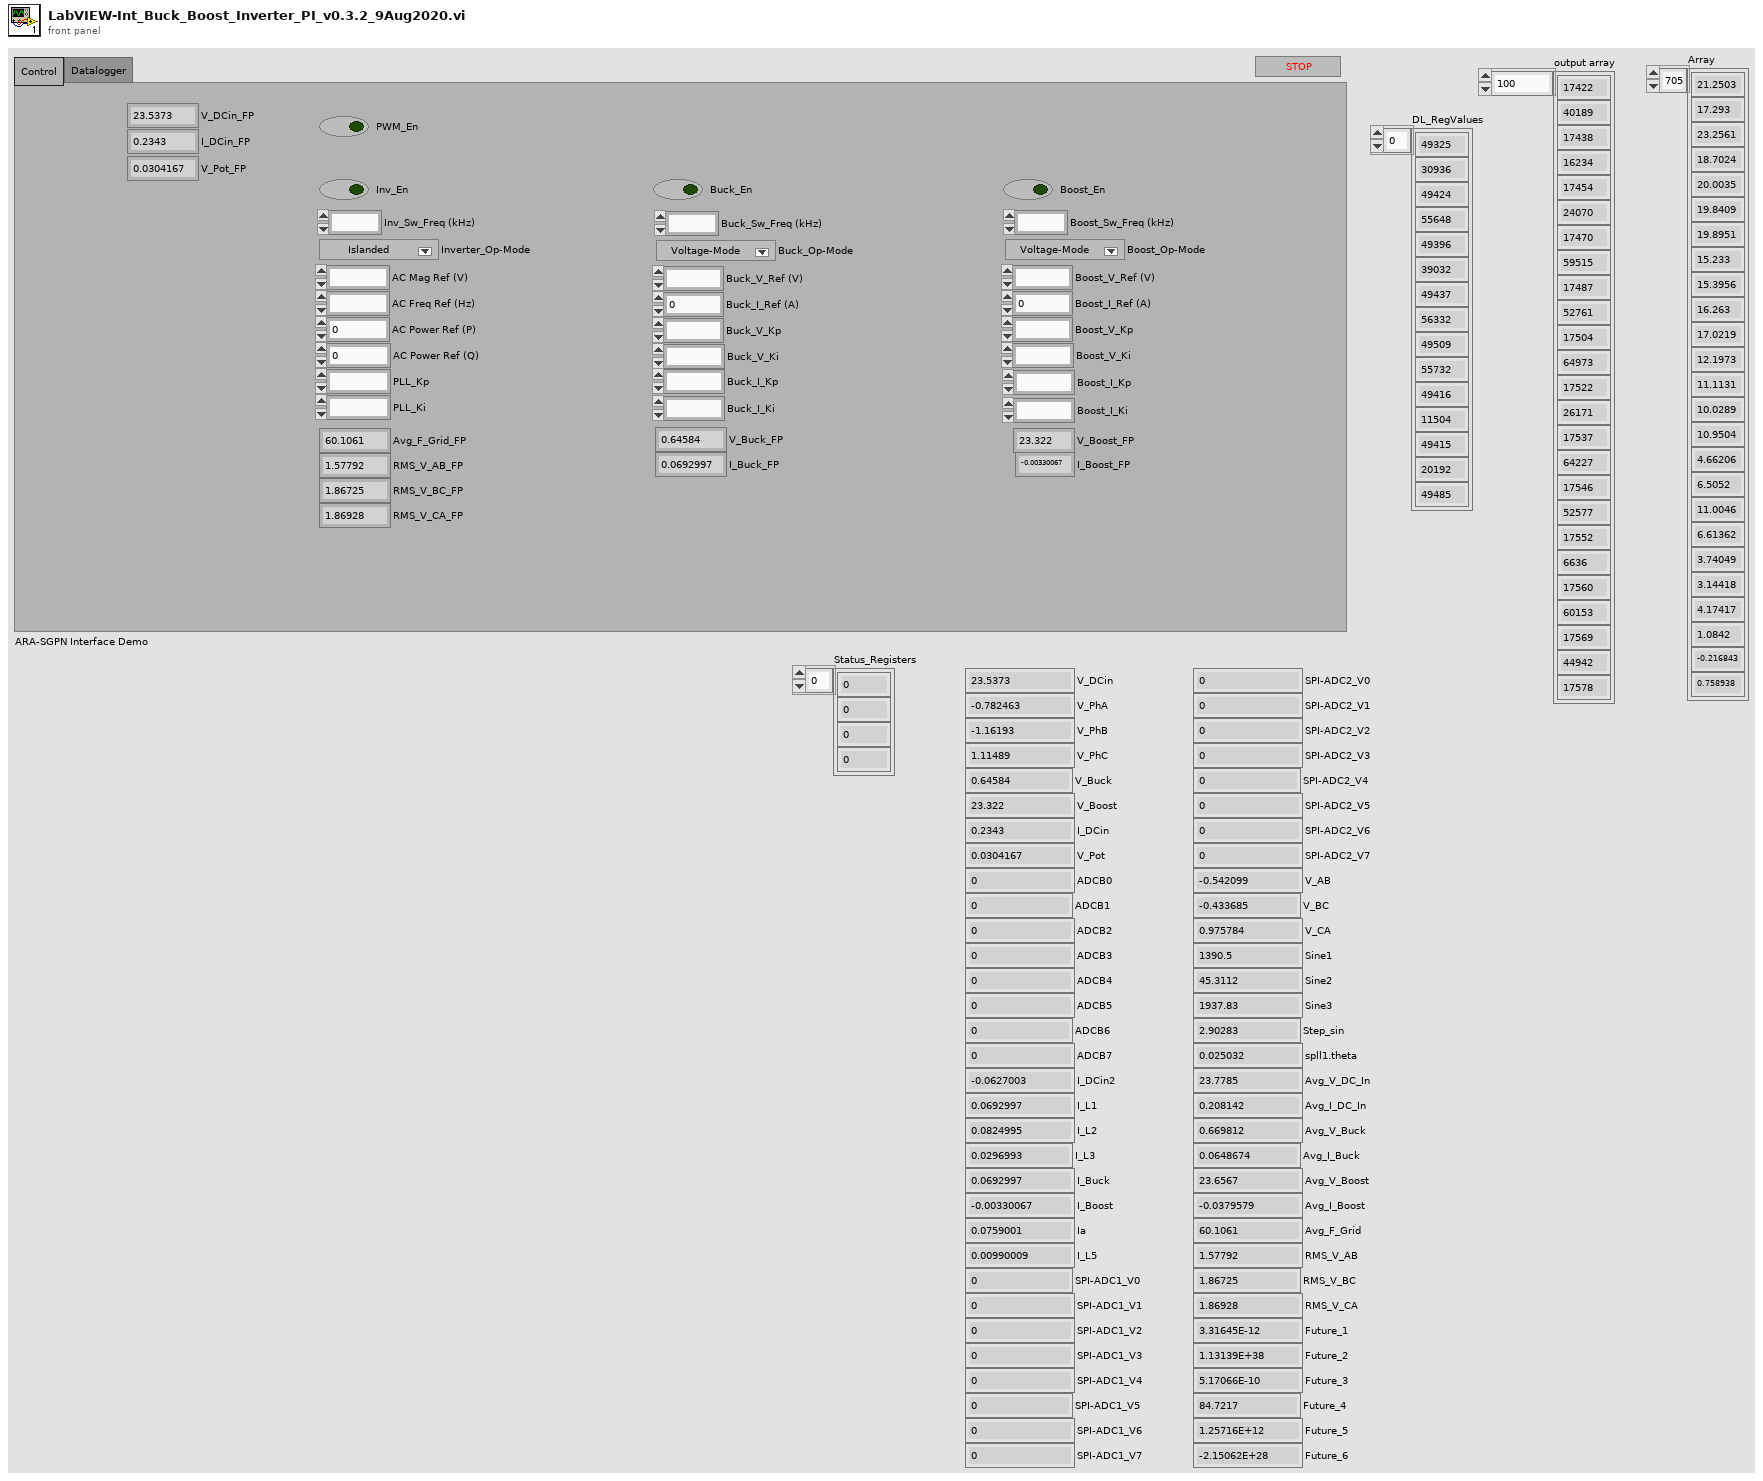
[diagram p1: front panel]
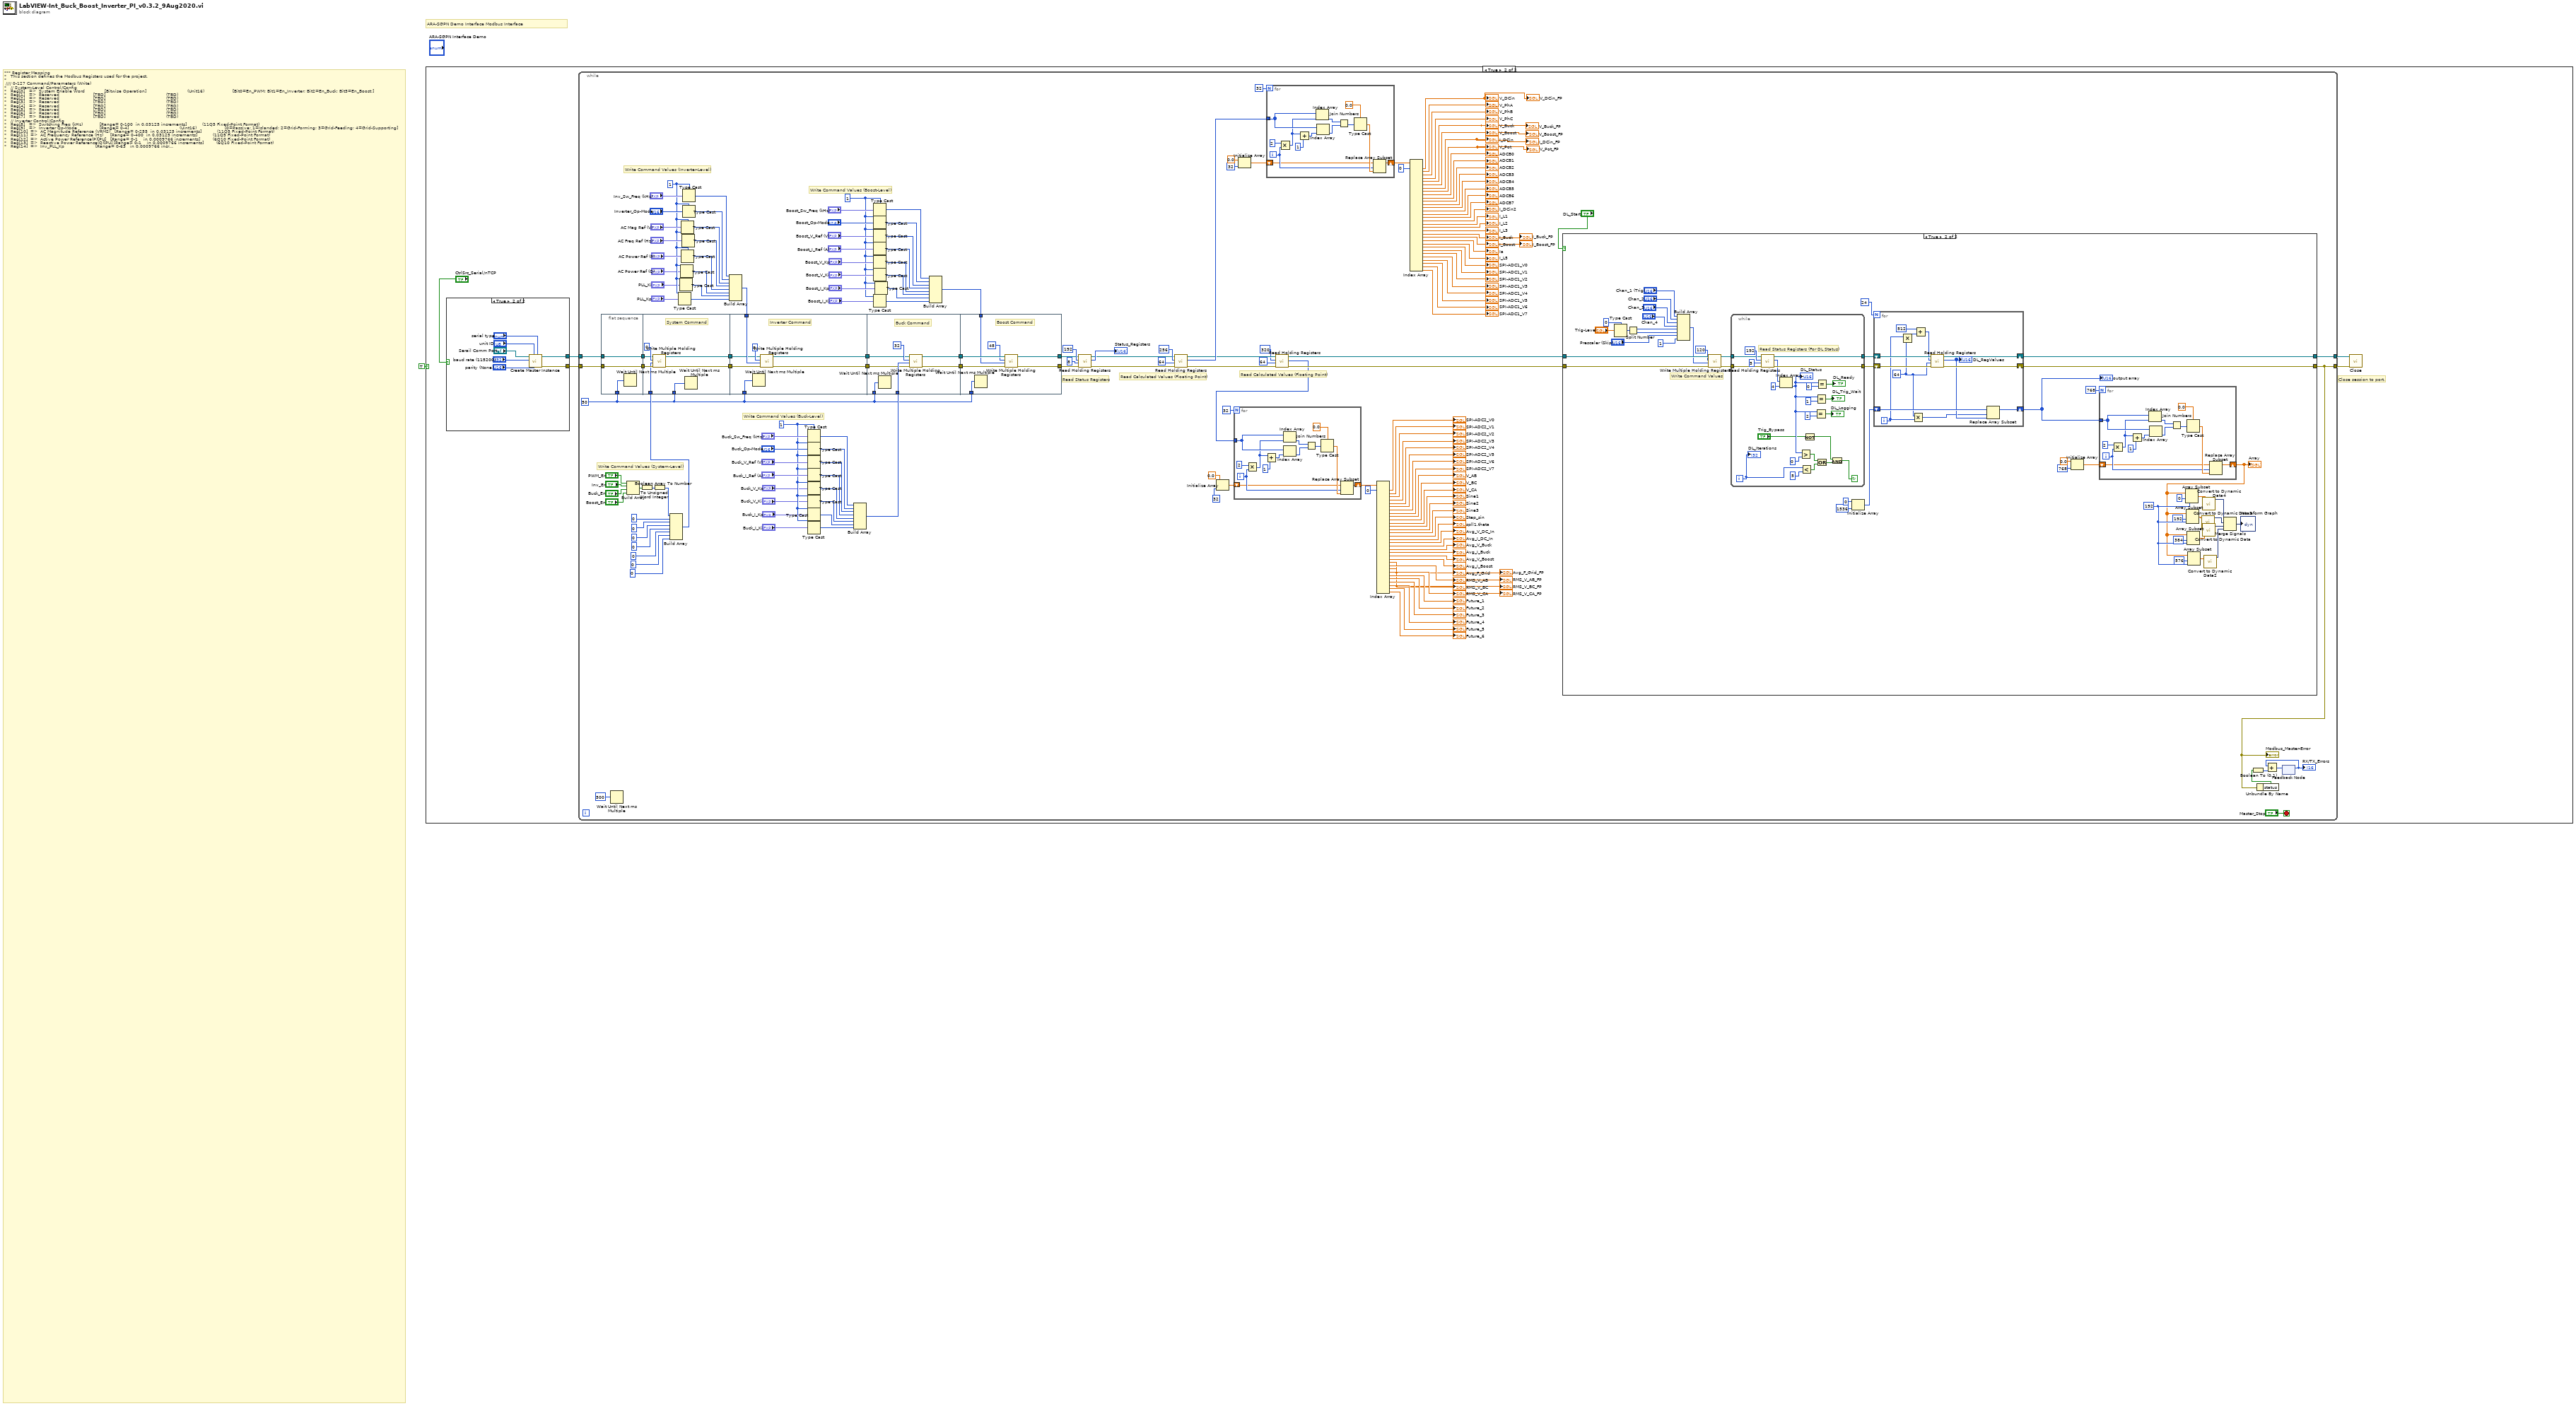
[diagram p0: block diagram]
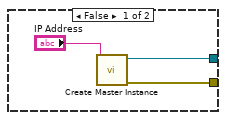
[diagram p3: hidden frame]
diagram:
  # "ARA-SGPN Demo Interface Modbus Interface"
  # "*** Register Mapping\n*   This section defines the Modbus Registers used for the project.\n*\n //// 0-127 Command/Parameters (Write)\n*   // System-Level Control/Config\n*   Reg[0]   =>  System Enable Word              [Bitwise Operation]                             (Unit16)                    [Bit0=En_PWM; Bit1=En_Inverter; Bit2=En_Buck; Bit3=En_Boost;]\n*   Reg[1]   =>  Reserved                        [TBD]                                           (TBD)\n*   Reg[2]   =>  Reserved                        [TBD]                                           (TBD)\n*   Reg[3]   =>  Reserved                        [TBD]                                           (TBD)\n*   Reg[4]   =>  Reserved                        [TBD]                                           (TBD)\n*   Reg[5]   =>  Reserved                        [TBD]                                           (TBD)\n*   Reg[6]   =>  Reserved                        [TBD]                                           (TBD)\n*   Reg[7]   =>  Reserved                        [TBD]                                           (TBD)\n*   // Inverter Control/Config\n*   Reg[8]   =>  Switching Freq (kHz)            [Range= 0-100  in 0.03125 increments]           (11Q5 Fixed-Point Format)\n*   Reg[9]   =>  Inverter Op-Mode                [Range= 0-4]                                    (Uint16)                    [0=Passive; 1=Islanded; 2=Grid-Forming; 3=Grid-Feeding; 4=Grid-Supporting]\n*   Reg[10]  =>  AC Magnitude Reference (VRMS)   [Range= 0-255  in 0.03125 increments]           (11Q5 Fixed-Point Format)\n*   Reg[11]  =>  AC Frequency Reference (Hz)     [Range= 0-400  in 0.03125 increments]           (11Q5 Fixed-Point Format)\n*   Reg[12]  =>  Active Power Reference(P)[PU]   [Range= 0-1    in 0.0009766 increments]         (6Q10 Fixed-Point Format)\n*   Reg[13]  =>  Reactive Power Reference(Q)[PU] [Range= 0-1    in 0.0009766 increments]         (6Q10 Fixed-Point Format)\n*   Reg[14]  =>  Inv_PLL_Kp                      [Range= 0-63   in 0.0009766 increments]         (6Q10 Fixed-Point Format)\n*   Reg[15]  =>  Inv_PLL_Ki                      [Range= 0-63   in 0.0009766 increments]         (6Q10 Fixed-Point Format)\n*   Reg[16]  =>  Reserved                        [Range= 0-63   in 0.0009766 increments]         (6Q10 Fixed-Point Format)\n*   Reg[17]  =>  Reserved                        [Range= 0-63   in 0.0009766 increments]         (6Q10 Fixed-Point Format)\n*   Reg[18]  =>  Reserved                        [Range= 0-63   in 0.0009766 increments]         (6Q10 Fixed-Point Format)\n*   Reg[19]  =>  Reserved                        [Range= 0-63   in 0.0009766 increments]         (6Q10 Fixed-Point Format)\n*   Reg[20]  =>  Reserved                        [Range= 0-63   in 0.0009766 increments]         (6Q10 Fixed-Point Format)\n*   Reg[21]  =>  Reserved                        [Range= 0-63   in 0.0009766 increments]         (6Q10 Fixed-Point Format)\n*   Reg[22]  =>  Reserved                        [Range= 0-63   in 0.0009766 increments]         (6Q10 Fixed-Point Format)\n*   Reg[23]  =>  Reserved                        [Range= 0-63   in 0.0009766 increments]         (6Q10 Fixed-Point Format)\n*   Reg[24]  =>  Reserved                        [Range= 0-63   in 0.0009766 increments]         (6Q10 Fixed-Point Format)\n*   Reg[25]  =>  Reserved                        [Range= 0-63   in 0.0009766 increments]         (6Q10 Fixed-Point Format)\n*   Reg[26]  =>  Reserved                        [Range= 0-63   in 0.0009766 increments]         (6Q10 Fixed-Point Format)\n*   Reg[27]  =>  Reserved                        [Range= 0-63   in 0.0009766 increments]         (6Q10 Fixed-Point Format)\n*   Reg[28]  =>  Reserved                        [Range= 0-63   in 0.0009766 increments]         (6Q10 Fixed-Point Format)\n*   Reg[29]  =>  Reserved                        [Range= 0-63   in 0.0009766 increments]         (6Q10 Fixed-Point Format)\n*   Reg[30]  =>  Reserved                        [Range= 0-63   in 0.0009766 increments]         (6Q10 Fixed-Point Format)\n*   Reg[31]  =>  Reserved                        [Range= 0-63   in 0.0009766 increments]         (6Q10 Fixed-Point Format)\n*   // Buck Control/Config\n*   Reg[32]  =>  Switching Freq (kHz)            [Range= 0-100  in 0.03125 increments]           (11Q5 Fixed-Point Format)\n*   Reg[33]  =>  Buck Op-Mode                    [Range= 0-4]                                    (Uint16)                    [0=Passive; 1=Voltage-Mode; 2=Current-Mode; 3=Dual-Loop]\n*   Reg[34]  =>  Buck Reference Voltage          [Range= 0-63   in 0.0009766 increments]         (6Q10 Fixed-Point Format)\n*   Reg[35]  =>  Buck Reference Current          [Range= 0-63   in 0.0009766 increments]         (6Q10 Fixed-Point Format)\n*   Reg[36]  =>  Buck_V_Kp                       [Range= 0-63   in 0.0009766 increments]         (6Q10 Fixed-Point Format)\n*   Reg[37]  =>  Buck_V_Ki                       [Range= 0-63   in 0.0009766 increments]         (6Q10 Fixed-Point Format)\n*   Reg[38]  =>  Buck_I_Kp                       [Range= 0-63   in 0.0009766 increments]         (6Q10 Fixed-Point Format)\n*   Reg[39]  =>  Buck_I_Ki                       [Range= 0-63   in 0.0009766 increments]         (6Q10 Fixed-Point Format)\n*   Reg[40]  =>  Reserved                        [Range= 0-63   in 0.0009766 increments]         (6Q10 Fixed-Point Format)\n*   Reg[41]  =>  Reserved                        [Range= 0-63   in 0.0009766 increments]         (6Q10 Fixed-Point Format)\n*   Reg[42]  =>  Reserved                        [Range= 0-63   in 0.0009766 increments]         (6Q10 Fixed-Point Format)\n*   Reg[43]  =>  Reserved                        [Range= 0-63   in 0.0009766 increments]         (6Q10 Fixed-Point Format)\n*   Reg[44]  =>  Reserved                        [Range= 0-63   in 0.0009766 increments]         (6Q10 Fixed-Point Format)\n*   Reg[45]  =>  Reserved                        [Range= 0-63   in 0.0009766 increments]         (6Q10 Fixed-Point Format)\n*   Reg[46]  =>  Reserved                        [Range= 0-63   in 0.0009766 increments]         (6Q10 Fixed-Point Format)\n*   Reg[47]  =>  Reserved                        [Range= 0-63   in 0.0009766 increments]         (6Q10 Fixed-Point Format)\n*   // Boost Control/Config\n*   Reg[48]  =>  Switching Freq (kHz)            [Range= 0-100  in 0.03125 increments]           (11Q5 Fixed-Point Format)\n*   Reg[49]  =>  Boost Op-Mode                   [Range= 0-4]                                    (Uint16)                    [0=Passive; 1=Voltage-Mode; 2=Current-Mode; 3=Dual-Loop]\n*   Reg[50]  =>  Boost Reference Voltage         [Range= 0-63   in 0.0009766 increments]         (6Q10 Fixed-Point Format)\n*   Reg[51]  =>  Boost Reference Current         [Range= 0-63   in 0.0009766 increments]         (6Q10 Fixed-Point Format)\n*   Reg[52]  =>  Boost_V_Kp                      [Range= 0-63   in 0.0009766 increments]         (6Q10 Fixed-Point Format)\n*   Reg[53]  =>  Boost_V_Ki                      [Range= 0-63   in 0.0009766 increments]         (6Q10 Fixed-Point Format)\n*   Reg[54]  =>  Boost_I_Kp                      [Range= 0-63   in 0.0009766 increments]         (6Q10 Fixed-Point Format)\n*   Reg[55]  =>  Boost_I_Ki                      [Range= 0-63   in 0.0009766 increments]         (6Q10 Fixed-Point Format)\n*   Reg[56]  =>  Reserved                        [Range= 0-63   in 0.0009766 increments]         (6Q10 Fixed-Point Format)\n*   Reg[57]  =>  Reserved                        [Range= 0-63   in 0.0009766 increments]         (6Q10 Fixed-Point Format)\n*   Reg[58]  =>  Reserved                        [Range= 0-63   in 0.0009766 increments]         (6Q10 Fixed-Point Format)\n*   Reg[59]  =>  Reserved                        [Range= 0-63   in 0.0009766 increments]         (6Q10 Fixed-Point Format)\n*   Reg[60]  =>  Reserved                        [Range= 0-63   in 0.0009766 increments]         (6Q10 Fixed-Point Format)\n*   Reg[61]  =>  Reserved                        [Range= 0-63   in 0.0009766 increments]         (6Q10 Fixed-Point Format)\n*   Reg[62]  =>  Reserved                        [Range= 0-63   in 0.0009766 increments]         (6Q10 Fixed-Point Format)\n*   Reg[63]  =>  Reserved                        [Range= 0-63   in 0.0009766 increments]         (6Q10 Fixed-Point Format)\n*   // Datalogger Control/Config\n*   Reg[120] =>  Datalogger Chan1 Input Select   [Range= 0-128 (Reg_FP [Max])]                   (Unit16)\n*   Reg[121] =>  Datalogger Chan2 Input Select   [Range= 0-128 (Reg_FP [Max])]                   (Unit16)\n*   Reg[122] =>  Datalogger Chan3 Input Select   [Range= 0-128 (Reg_FP [Max])]                   (Unit16)\n*   Reg[123] =>  Datalogger Chan4 Input Select   [Range= 0-128 (Reg_FP [Max])]                   (Unit16)\n*   Reg[124] =>  Datalogger Chan1 Trigger (High) [Range= Floating Point]                         (Upper Portion of Float32)\n*   Reg[125] =>  Datalogger Chan1 Trigger (Low)  [Range= Floating Point]                         (Lower Portion of Float32)\n*   Reg[126] =>  Datalogger Prescaler            [Range= 0-65535 (Skip Count)]                   (Unit16)\n*   Reg[127] =>  Datalogger Start                [Flag to Start Logging; 1=Start]                (Unit16)\n*\n*\n*   //// 128-191 Raw ADC Data (Read) (Uint16)\n*   // DSP ADC_A\n*   Reg[128] => ADC_A0          (DC Input Voltage)          [PE-Eval PCB]\n*   Reg[129] => ADC_A1          (VAC_PhA Output Voltage)    [PE-Eval PCB]\n*   Reg[130] => ADC_A2          (VAC_PhB Output Voltage)    [PE-Eval PCB]\n*   Reg[131] => ADC_A3          (VAC_PhC Output Voltage)    [PE-Eval PCB]\n*   Reg[132] => ADC_A4          (V_Buck or DC_Link)         [PE-Eval PCB]       (Based on JP4 Position)\n*   Reg[133] => ADC_A5          (Boost Output Voltage)      [PE-Eval PCB]\n*   Reg[134] => ADC_A6          (DC Input Current)          [PE-Eval PCB]       (3V Scaling)\n*   Reg[135] => ADC_A7          (Potentiometer)             [PE-Eval PCB]       (3V Scaling)\n*   // DSP ADC_B\n*   Reg[136] => ADC_B0          (Not Used)\n*   Reg[137] => ADC_B1          (Not Used)\n*   Reg[138] => ADC_B2          (Not Used)\n*   Reg[139] => ADC_B3          (Not Used)\n*   Reg[140] => ADC_B4          (Not Used)\n*   Reg[141] => ADC_B5          (Not Used)\n*   Reg[142] => ADC_B6          (Not Used)\n*   Reg[143] => ADC_B7          (Not Used)\n*   // SPI ADC_0 (SPI-ADC on PE-Eval_vv1.6a)\n*   Reg[144] => SPI_ADC0_0      (DC Input Current)          [PE-Eval PCB]       (5V Scaling)\n*   Reg[145] => SPI_ADC0_1      (I_L1)                      [PE-Eval PCB]\n*   Reg[146] => SPI_ADC0_2      (I_L2)                      [PE-Eval PCB]\n*   Reg[147] => SPI_ADC0_3      (I_L3)                      [PE-Eval PCB]\n*   Reg[148] => SPI_ADC0_4      (I_Buck)                    [PE-Eval PCB]\n*   Reg[149] => SPI_ADC0_5      (I_Boost)                   [PE-Eval PCB]\n*   Reg[150] => SPI_ADC0_6      (Ia or I_L4)                [PE-Eval PCB]       (Based on JP3 Position)\n*   Reg[151] => SPI_ADC0_7      (I_L5)                      [PE-Eval PCB]\n*   // SPI ADC_1 (SPI-ADC IDC_C on UCB_v1.4a) [Not Used for this Project]\n*   Reg[152] => SPI_ADC1_0      (Not Used)\n*   Reg[153] => SPI_ADC1_1      (Not Used)\n*   Reg[154] => SPI_ADC1_2      (Not Used)\n*   Reg[155] => SPI_ADC1_3      (Not Used)\n*   Reg[156] => SPI_ADC1_4      (Not Used)\n*   Reg[157] => SPI_ADC1_5      (Not Used)\n*   Reg[158] => SPI_ADC1_6      (Not Used)\n*   Reg[159] => SPI_ADC1_7      (Not Used)\n*   // SPI ADC_2 (SPI-ADC IDC_D on UCB_v1.4a) [Not Used for this Project]\n*   Reg[160] => SPI_ADC2_0      (Not Used)\n*   Reg[161] => SPI_ADC2_1      (Not Used)\n*   Reg[162] => SPI_ADC2_2      (Not Used)\n*   Reg[163] => SPI_ADC2_3      (Not Used)\n*   Reg[164] => SPI_ADC2_4      (Not Used)\n*   Reg[165] => SPI_ADC2_5      (Not Used)\n*   Reg[166] => SPI_ADC2_6      (Not Used)\n*   Reg[167] => SPI_ADC2_7      (Not Used)\n*\n*\n*   //// 192-255 Status and Information (Read) (Uint16)\n*   Reg[192]    => Status Word 1        // General Information (Future Use)\n*   Reg[193]    => Status Word 2        // General Information (Future Use)\n*   Reg[194]    => Status Word 3        // General Information (Future Use)\n*   Reg[195]    => Status Word 4        // General Information (Future Use)\n*   Reg[196]    => DL_Status            // Datalogger Status [1 = Waiting Trigger; 2=Collecting;]\n*\n*   //// 256-511 Calculated Parameters (Read)      128 Entries(32-Bit Floating Point) [Upper then Lower using Datacon.F_Data]\n*   // Maps to Reg_FP[] Floating Point Array Referenced Below\n*   DataCon.F_Data = Reg_FP[x];\n*   mb.holdingRegisters.Mod_Reg[(i*2)+256] = DataCon.Reg_Data[1];   //Upper Word of Float\n*   mb.holdingRegisters.Mod_Reg[(i*2)+257] = DataCon.Reg_Data[0];   //Lower Word of Float\n*\n*   // DSP-ADC_A Values Scaled and Converted to Floating Point Representation (Inverter)\n*   Reg_FP[0] = V_DCin;\n*   Reg_FP[1] = V_PhA;\n*   Reg_FP[2] = V_PhB;\n*   Reg_FP[3] = V_PhC;\n*   Reg_FP[4] = V_Buck;\n*   Reg_FP[5] = V_Boost;\n*   Reg_FP[6] = I_DCin;\n*   Reg_FP[7]=  V_Pot;\n*   // DSP-ADC_B Values Scaled and Converted to Floating Point Representation (Future Use)\n*   Reg_FP[8]=  0;                  //Future Use (ADCB0)\n*   Reg_FP[9]=  0;                  //Future Use (ADCB1)\n*   Reg_FP[10]=  0;                 //Future Use (ADCB2)\n*   Reg_FP[11]=  0;                 //Future Use (ADCB3)\n*   Reg_FP[12]=  0;                 //Future Use (ADCB4)\n*   Reg_FP[13]=  0;                 //Future Use (ADCB5)\n*   Reg_FP[14]=  0;                 //Future Use (ADCB6)\n*   Reg_FP[15]=  0;                 //Future Use (ADCB7)\n*   // SPI-ADC_0 Values Scaled and Converted to Floating Point Representation (PE-Eval PCB)\n*   Reg_FP[16]= I_DCin2;            //Updated in SPI Interrupt\n*   Reg_FP[17]= I_L1;               //Updated in SPI Interrupt\n*   Reg_FP[18]= I_L2;               //Updated in SPI Interrupt\n*   Reg_FP[19]= I_L3;               //Updated in SPI Interrupt\n*   Reg_FP[20]=I_Buck;              //Updated in SPI Interrupt\n*   Reg_FP[21]=I_Boost;             //Updated in SPI Interrupt\n*   Reg_FP[22]=Ia;                  //Updated in SPI Interrupt\n*   Reg_FP[23]=I_L5;                //Updated in SPI Interrupt\n*   // SPI-ADC_1 Values Scaled and Converted to Floating Point Representation (Future Use)\n*   Reg_FP[24]= 0;                  //Future Use (SPI-ADC_1-V0)\n*   Reg_FP[25]= 0;                  //Future Use (SPI-ADC_1-V1)\n*   Reg_FP[26]= 0;                  //Future Use (SPI-ADC_1-V2)\n*   Reg_FP[27]= 0;                  //Future Use (SPI-ADC_1-V3)\n*   Reg_FP[28]= 0;                  //Future Use (SPI-ADC_1-V4)\n*   Reg_FP[29]= 0;                  //Future Use (SPI-ADC_1-V5)\n*   Reg_FP[30]= 0;                  //Future Use (SPI-ADC_1-V6)\n*   Reg_FP[31]= 0;                  //Future Use (SPI-ADC_1-V7)\n*   // SPI-ADC_2 Values Scaled and Converted to Floating Point Representation (Future Use)\n*   Reg_FP[32]= 0;                  //Future Use (SPI-ADC_2-V0)\n*   Reg_FP[33]= 0;                  //Future Use (SPI-ADC_2-V1)\n*   Reg_FP[34]= 0;                  //Future Use (SPI-ADC_2-V2)\n*   Reg_FP[35]= 0;                  //Future Use (SPI-ADC_2-V3)\n*   Reg_FP[36]= 0;                  //Future Use (SPI-ADC_2-V4)\n*   Reg_FP[37]= 0;                  //Future Use (SPI-ADC_2-V5)\n*   Reg_FP[38]= 0;                  //Future Use (SPI-ADC_2-V6)\n*   Reg_FP[39]= 0;                  //Future Use (SPI-ADC_2-V7)\n*   // Calculated Values\n*   Reg_FP[40] = V_AB;\n*   Reg_FP[41] = V_BC;\n*   Reg_FP[42] = V_CA;\n*   Reg_FP[43] = Sine1;\n*   Reg_FP[44] = Sine2;\n*   Reg_FP[45] = Sine3;\n*   Reg_FP[46] = Step_sin;\n*   Reg_FP[47] = spll1.theta[0];\n*   // Average and RMS Values\n*   Reg_FP[48] = Avg_V_DC_In;\n*   Reg_FP[49] = Avg_I_DC_In;\n*   Reg_FP[50] = Avg_V_Buck;\n*   Reg_FP[51] = Avg_I_Buck;\n*   Reg_FP[52] = Avg_V_Boost;\n*   Reg_FP[53] = Avg_I_Boost;\n*   Reg_FP[54] = Avg_F_Grid;\n*   Reg_FP[55] = RMS_V_AB;\n*   Reg_FP[56] = RMS_V_BC;\n*   Reg_FP[57] = RMS_V_CA;\n*\n*   //// 512-2047 Datalogging              4-Channels with 192 Floating Point values per channel (32-Bit Floating Point) [Upper then Lower using Datacon.F_Data]\n*   Reg[512-895]    => Channel_1        Channel_1 Data\n*   Reg[896-1279]   => Channel_2        Channel_2 Data\n*   Reg[1280-1663]  => Channel_3        Channel_3 Data\n*   Reg[1664-2047]  => Channel_4        Channel_4 Data"
  n1 = case shown="True" TRUE {
    frame False {
    }
    frame True {
      # "Close session to port."
      n2 = case shown="True" "CtrlSrc_Serial/nTCP" {
        tunnel: [w7 w11] -> w4
        tunnel: [w8 w10] -> w3
        frame False {
          n3 = call-poly <vilib>:"Create Master Instance.vi"("address"="IP Address") -> ("error out"=w7:errorcluster, "TCP master instance"=w8:refnum<class "Modbus Master.lvclass">)  [unwired: 9 in]
        }
        frame True {
          n4 = call-poly <vilib>:"Create Master Instance.vi"("serial type"="serial type", "parity (Even)"="parity (None)", "unit ID"="unit ID", "baud rate (9600)"="baud rate (115200)", "VISA resource name"="Serail Comm Port") -> ("error out"=w11:errorcluster, "serial master instance"=w10:refnum<class "Modbus Master.lvclass">)  [unwired: 5 in]
        }
      }
      n5 = while {
        tunnel: [w177] -> w6
        tunnel: [w178] -> w5
        tunnel: w4 -> [w68]
        tunnel: w3 -> [w67]
        stop <- "Master_Stop" stop-if-true
        w31 = u16 1 ("starting address")
        w48 = u32 50
        w108 = u16 1 ("starting address")
        w180 = u16 1 ("starting address")
        # "Write Command Values (Boost-Level)"
        # "Read Status Registers"
        # "Read Calculated Values (Floating Point)"
        # "Read Calculated Values (Floating Point)"
        # "Write Command Values (Buck-Level)"
        # "Write Command Values (Inverter-Level)"
        # "Write Command Values (System-Level)"
        n6 = flat-sequence {
          tunnel: w67 -> [w213]
          tunnel: w68 -> [w214]
          tunnel: [w214] -> w51
          tunnel: [w213] -> w50
          tunnel: w48 -> [w212]
          tunnel: [w218] -> w61
          tunnel: [w217] -> w56
          tunnel: w48 -> [w216]
          tunnel: w51 -> [w221]
          tunnel: w50 -> [w219]
          tunnel: w49 -> [w215]
          tunnel: w63 -> [w228]
          tunnel: w61 -> [w226]
          tunnel: [w225] -> w60
          tunnel: w56 -> [w224]
          tunnel: [w223] -> w55
          tunnel: w48 -> [w222]
          tunnel: w62 -> [w235]
          tunnel: w60 -> [w233]
          tunnel: [w232] -> w59
          tunnel: w55 -> [w231]
          tunnel: [w230] -> w54
          tunnel: w48 -> [w229]
          tunnel: w59 -> [w240]
          tunnel: [w238] -> w58
          tunnel: w54 -> [w241]
          tunnel: [w239] -> w53
          tunnel: w48 -> [w242]
          tunnel: w39 -> [w237]
          frame #0 {
            n7 = Wait Until Next ms Multiple(millisecond multiple=w212) -> ()  [unwired: 1 out]
          }
          frame #1 {
            # "System Command"
            n8 = call-dynamic "Write Multiple Holding Registers.vi"("error in (no error)"=w221, "holding register values"=w215, "starting address"=u16 0, "Modbus master in"=w219) -> ("error out"=w218:errorcluster, "Modbus master out"=w217:refnum<class "Modbus Master.lvclass">)  [unwired: 6 in]
            n9 = Wait Until Next ms Multiple(millisecond multiple=w216) -> ()  [unwired: 1 out]
          }
          frame #2 {
            # "Inverter Command"
            n10 = Wait Until Next ms Multiple(millisecond multiple=w222) -> ()  [unwired: 1 out]
            n11 = call-dynamic "Write Multiple Holding Registers.vi"("error in (no error)"=w226, "holding register values"=w228, "starting address"=u16 8, "Modbus master in"=w224) -> ("error out"=w225:errorcluster, "Modbus master out"=w223:refnum<class "Modbus Master.lvclass">)  [unwired: 6 in]
          }
          frame #3 {
            # "Buck Command"
            n12 = Wait Until Next ms Multiple(millisecond multiple=w229) -> ()  [unwired: 1 out]
            n13 = call-dynamic "Write Multiple Holding Registers.vi"("error in (no error)"=w233, "holding register values"=w235, "starting address"=u16 32, "Modbus master in"=w231) -> ("error out"=w232:errorcluster, "Modbus master out"=w230:refnum<class "Modbus Master.lvclass">)  [unwired: 6 in]
          }
          frame #4 {
            # "Boost Command"
            n14 = Wait Until Next ms Multiple(millisecond multiple=w242) -> ()  [unwired: 1 out]
            n15 = call-dynamic "Write Multiple Holding Registers.vi"("error in (no error)"=w240, "holding register values"=w237, "starting address"=u16 48, "Modbus master in"=w241) -> ("error out"=w238:errorcluster, "Modbus master out"=w239:refnum<class "Modbus Master.lvclass">)  [unwired: 6 in]
          }
        }
        n16 = Wait Until Next ms Multiple(millisecond multiple=u32 500) -> ()  [unwired: 1 out]
        n17 = Build Array("PWM_En", "Inv_En", "Buck_En", "Boost_En") -> (w160:bool[])
        n18 = Boolean Array To Number(Boolean array=w160) -> (number=w159:u32)
        n19 = To Unsigned Word Integer(number=w159) -> (unsigned 16bit integer=w175:u16)
        n20 = Build Array(w175, u16 0 ("element"), u16 0 ("element"), u16 0 ("element"), u16 0 ("element"), u16 0 ("element"), u16 0 ("element"), u16 0 ("element")) -> (w49:u16[])
        n21 = Type Cast(type=w180, x="PLL_Kp") -> (*(type *) &x=w189:u16)
        n22 = Type Cast(type=w180, x="PLL_Ki") -> (*(type *) &x=w190:u16)
        n23 = Type Cast(type=w180, x="AC Power Ref (Q)") -> (*(type *) &x=w191:u16)
        n24 = Type Cast(type=w180, x="AC Power Ref (P)") -> (*(type *) &x=w183:u16)
        n25 = Type Cast(type=w180, x="AC Mag Ref (V)") -> (*(type *) &x=w187:u16)
        n26 = Type Cast(type=w180, x="AC Freq Ref (Hz)") -> (*(type *) &x=w184:u16)
        n27 = Type Cast(type=w180, x="Inverter_Op-Mode") -> (*(type *) &x=w188:u16)
        n28 = Type Cast(type=w180, x="Inv_Sw_Freq (kHz)") -> (*(type *) &x=w182:u16)
        n29 = Build Array(w182, w188, w187, w184, w183, w191, w190, w189) -> (w63:u16[])
        n30 = Type Cast(type=w108, x="Buck_Sw_Freq (kHz)") -> (*(type *) &x=w112:u16)
        n31 = Type Cast(type=w108, x="Buck_Op-Mode") -> (*(type *) &x=w117:u16)
        n32 = Type Cast(type=w108, x="Buck_V_Ref (V)") -> (*(type *) &x=w116:u16)
        n33 = Type Cast(type=w108, x="Buck_I_Ref (A)") -> (*(type *) &x=w114:u16)
        n34 = Type Cast(type=w108, x="Buck_V_Kp") -> (*(type *) &x=w113:u16)
        n35 = Type Cast(type=w108, x="Buck_V_Ki") -> (*(type *) &x=w120:u16)
        n36 = Type Cast(type=w108, x="Buck_I_Kp") -> (*(type *) &x=w119:u16)
        n37 = Type Cast(type=w108, x="Buck_I_Ki") -> (*(type *) &x=w118:u16)
        n38 = Build Array(w112, w117, w116, w114, w113, w120, w119, w118) -> (w62:u16[])
        n39 = Type Cast(type=w31, x="Boost_Sw_Freq (kHz)") -> (*(type *) &x=w38:u16)
        n40 = Type Cast(type=w31, x="Boost_Op-Mode") -> (*(type *) &x=w37:u16)
        n41 = Type Cast(type=w31, x="Boost_V_Ref (V)") -> (*(type *) &x=w36:u16)
        n42 = Type Cast(type=w31, x="Boost_I_Ref (A)") -> (*(type *) &x=w35:u16)
        n43 = Type Cast(type=w31, x="Boost_V_Kp") -> (*(type *) &x=w34:u16)
        n44 = Type Cast(type=w31, x="Boost_V_Ki") -> (*(type *) &x=w33:u16)
        n45 = Type Cast(type=w31, x="Boost_I_Ki") -> (*(type *) &x=w45:u16)
        n46 = Type Cast(type=w31, x="Boost_I_Kp") -> (*(type *) &x=w30:u16)
        n47 = Build Array(w38, w37, w36, w35, w34, w33, w30, w45) -> (w39:u16[])
        n48 = call-dynamic "Read Holding Registers.vi"("error in (no error)"=w58, "number of holding registers"=u16 8, "starting address"=u16 192, "Modbus master in"=w53) -> ("error out"=w57:errorcluster, "register values"=→"Status_Registers":u16[], "Modbus master out"=w52:refnum<class "Modbus Master.lvclass">)  [unwired: 5 in]
        n49 = call-dynamic "Read Holding Registers.vi"("error in (no error)"=w57, "number of holding registers"=u16 64 ("starting address"), "starting address"=u16 256, "Modbus master in"=w52) -> ("error out"=w126:errorcluster, "register values"=w154:u16[], "Modbus master out"=w125:refnum<class "Modbus Master.lvclass">)  [unwired: 5 in]
        n50 = Initialize Array(sgl 0.0 ("element"), 32 ("dimension size")) -> (w100:sgl[])
        n51 = Initialize Array(sgl 0.0 ("element"), 32 ("dimension size")) -> (w155:sgl[])
        n52 = for {
          N: 32 -> [_]
          tunnel: w154 -> [w255]
          shift-right: [w244] -> w153
          shift-left: w155 -> [w243]
          i -> [w245]
          n53 = Multiply(x=2, y=w245) -> (x*y=w253:i32)
          n54 = Add(x=w253, y=1) -> (x+y=w251:i32)
          n55 = Index Array(array=w255, index=w253) -> (element=w249:u16)
          n56 = Index Array(array=w255, index=w251) -> (element=w250:u16)
          n57 = Join Numbers(hi=w249, lo=w250) -> ((hi.lo)=w248:u32)
          n58 = Type Cast(type=sgl 0.0 ("y"), x=w248) -> (*(type *) &x=w246:sgl)
          n59 = Replace Array Subset(array=w243, new element=w246, index=w245) -> (w244:sgl[])
        }
        n60 = call-dynamic "Read Holding Registers.vi"("error in (no error)"=w126, "number of holding registers"=u16 64 ("starting address"), "starting address"=u16 320, "Modbus master in"=w125) -> ("error out"=w123:errorcluster, "register values"=w99:u16[], "Modbus master out"=w124:refnum<class "Modbus Master.lvclass">)  [unwired: 5 in]
        n61 = for {
          N: 32 -> [_]
          tunnel: w99 -> [w211]
          shift-right: [w200] -> w98
          shift-left: w100 -> [w199]
          i -> [w201]
          n62 = Multiply(x=2, y=w201) -> (x*y=w209:i32)
          n63 = Add(x=w209, y=1) -> (x+y=w207:i32)
          n64 = Index Array(array=w211, index=w209) -> (element=w205:u16)
          n65 = Index Array(array=w211, index=w207) -> (element=w206:u16)
          n66 = Join Numbers(hi=w205, lo=w206) -> ((hi.lo)=w204:u32)
          n67 = Type Cast(type=sgl 0.0 ("y"), x=w204) -> (*(type *) &x=w202:sgl)
          n68 = Replace Array Subset(array=w199, new element=w202, index=w201) -> (w200:sgl[])
        }
        n69 = Index Array(array=w98, index #1=0 ("index")) -> (element #1=→"SPI-ADC2_V0":sgl, element #2=→"SPI-ADC2_V1":sgl, element #3=→"SPI-ADC2_V2":sgl, element #4=→"SPI-ADC2_V3":sgl, element #5=→"SPI-ADC2_V4":sgl, element #6=→"SPI-ADC2_V5":sgl, element #7=→"SPI-ADC2_V6":sgl, element #8=→"SPI-ADC2_V7":sgl, element #9=→"V_AB":sgl, element #10=→"V_BC":sgl, element #11=→"V_CA":sgl, element #12=→"Sine1":sgl, element #13=→"Sine2":sgl, element #14=→"Sine3":sgl, element #15=→"Step_sin":sgl, element #16=→"spll1.theta":sgl, element #17=→"Avg_V_DC_In":sgl, element #18=→"Avg_I_DC_In":sgl, element #19=→"Avg_V_Buck":sgl, element #20=→"Avg_I_Buck":sgl, element #21=→"Avg_V_Boost":sgl, element #22=→"Avg_I_Boost":sgl, element #23=→"Avg_F_Grid" →"Avg_F_Grid_FP":sgl, element #24=→"RMS_V_AB" →"RMS_V_AB_FP":sgl, element #25=→"RMS_V_BC" →"RMS_V_BC_FP":sgl, element #26=→"RMS_V_CA" →"RMS_V_CA_FP":sgl, element #27=→"Future_1":sgl, element #28=→"Future_2":sgl, element #29=→"Future_3":sgl, element #30=→"Future_4":sgl, element #31=→"Future_5":sgl, element #32=→"Future_6":sgl)  [unwired: 31 in]
        n70 = Index Array(array=w153, index #1=0 ("index")) -> (element #1=→"V_DCin" →"V_DCin_FP":sgl, element #2=→"V_PhA":sgl, element #3=→"V_PhB":sgl, element #4=→"V_PhC":sgl, element #5=→"V_Buck" →"V_Buck_FP":sgl, element #6=→"V_Boost" →"V_Boost_FP":sgl, element #7=→"I_DCin" →"I_DCin_FP":sgl, element #8=→"V_Pot" →"V_Pot_FP":sgl, element #9=→"ADCB0":sgl, element #10=→"ADCB1":sgl, element #11=→"ADCB2":sgl, element #12=→"ADCB3":sgl, element #13=→"ADCB4":sgl, element #14=→"ADCB5":sgl, element #15=→"ADCB6":sgl, element #16=→"ADCB7":sgl, element #17=→"I_DCin2":sgl, element #18=→"I_L1":sgl, element #19=→"I_L2":sgl, element #20=→"I_L3":sgl, element #21=→"I_Buck" →"I_Buck_FP":sgl, element #22=→"I_Boost" →"I_Boost_FP":sgl, element #23=→"Ia":sgl, element #24=→"I_L5":sgl, element #25=→"SPI-ADC1_V0":sgl, element #26=→"SPI-ADC1_V1":sgl, element #27=→"SPI-ADC1_V2":sgl, element #28=→"SPI-ADC1_V3":sgl, element #29=→"SPI-ADC1_V4":sgl, element #30=→"SPI-ADC1_V5":sgl, element #31=→"SPI-ADC1_V6":sgl, element #32=→"SPI-ADC1_V7":sgl)  [unwired: 31 in]
        n71 = case shown="True" "DL_Start" {
          tunnel: [w257 w302] -> w178
          tunnel: [w256 w301] -> w177
          tunnel: w123 -> [w256 w300]
          tunnel: w124 -> [w257 w299]
          frame False {
          }
          frame True {
            w278 = 192 ("length")
            # "Write Command Values"
            n72 = Type Cast(type=u32 0 ("starting address"), x="Trig-Level") -> (*(type *) &x=w293:u32)
            n73 = Split Number(x=w293) -> (hi(x)=w295:u16, lo(x)=w294:u16)
            n74 = Build Array("Chan_1 (Trig)", "Chan_2", "Chan_3", "Chan_4", w295, w294, "Prescaler (Skip)", u16 1 ("starting address")) -> (w297:u16[])
            n75 = call-dynamic "Write Multiple Holding Registers.vi"("error in (no error)"=w300, "holding register values"=w297, "starting address"=u16 120, "Modbus master in"=w299) -> ("error out"=w262:errorcluster, "Modbus master out"=w264:refnum<class "Modbus Master.lvclass">)  [unwired: 6 in]
            n76 = while {
              tunnel: w262 -> [w321]
              tunnel: [w320] -> w261
              tunnel: w264 -> [w323]
              tunnel: [w322] -> w263
              i -> [w315]
              stop <- w303 continue-if-true
              # "Read Status Registers (For DL Status)"
              n77 = call-dynamic "Read Holding Registers.vi"("error in (no error)"=w321, "number of holding registers"=u16 5, "starting address"=u16 192, "Modbus master in"=w323) -> ("error out"=w320:errorcluster, "register values"=w314:u16[], "Modbus master out"=w322:refnum<class "Modbus Master.lvclass">)  [unwired: 5 in]
              n78 = Index Array(array=w314, index=4) -> (element=w313:u16)
              "DL_Status" <- w313
              n79 = Greater?(x=w313, y=u16 0) -> (0:w318:bool)
              n80 = Less?(x=w315, y=5) -> (x < y?=w316:bool)
              n81 = Not(x="Trig_Bypass") -> (.not. x?=w304:bool)
              n82 = Equal?(x=w313, y=u16 2) -> (x = y?=→"DL_Logging":bool)
              n83 = Equal?(x=w313, y=u16 1) -> (x = y?=→"DL_Trig_Wait":bool)
              n84 = Equal?(x=w313, y=u16 0) -> (x = y?=→"DL_Ready":bool)
              n85 = Or(x=w318, y=w316) -> (x .or. y?=w306:bool)
              n86 = And(x=w304, y=w306) -> (x .and. y?=w303:bool)
              "DL_Iterations" <- w315
            }
            n87 = Initialize Array(u16 0 ("element"), 1536 ("dimension size")) -> (w285:u16[])
            n88 = for {
              N: 24 -> [_]
              shift-right: [w350] -> w301
              shift-left: w261 -> [w352]
              shift-right: [w351] -> w302
              shift-left: w263 -> [w349]
              shift-right: [w345] -> w283
              shift-left: w285 -> [w344]
              i -> [w342]
              w343 = u16 64 ("number of holding registers")
              n89 = Multiply(x=w342, y=w343) -> (x*y=w347:i32)
              n90 = Multiply(x=w343, y=w342) -> (x*y=w340:i32)
              n91 = Add(x=u16 512 ("starting address"), y=w347) -> (x+y=w346:i32)
              n92 = call-dynamic "Read Holding Registers.vi"("error in (no error)"=w352, "number of holding registers"=w343, "starting address"=w346, "Modbus master in"=w349) -> ("error out"=w350:errorcluster, "register values"=w341:u16[], "Modbus master out"=w351:refnum<class "Modbus Master.lvclass">)  [unwired: 5 in]
              "DL_RegValues" <- w341
              n93 = Replace Array Subset(array=w344, new element=w341, index=w340) -> (w345:u16[])
            }
            "output array" <- w283
            n94 = Initialize Array(sgl 0.0 ("element"), 768 ("dimension size")) -> (w280:sgl[])
            n95 = for {
              N: 768 -> [_]
              tunnel: w283 -> [w339]
              shift-right: [w328] -> w266
              shift-left: w280 -> [w327]
              i -> [w329]
              n96 = Multiply(x=2, y=w329) -> (x*y=w337:i32)
              n97 = Add(x=w337, y=1) -> (x+y=w335:i32)
              n98 = Index Array(array=w339, index=w337) -> (element=w333:u16)
              n99 = Index Array(array=w339, index=w335) -> (element=w334:u16)
              n100 = Join Numbers(hi=w333, lo=w334) -> ((hi.lo)=w332:u32)
              n101 = Type Cast(type=sgl 0.0 ("y"), x=w332) -> (*(type *) &x=w330:sgl)
              n102 = Replace Array Subset(array=w327, new element=w330, index=w329) -> (w328:sgl[])
            }
            "Array" <- w266
            n103 = Array Subset(array=w266, index=0, length=w278) -> (w268:sgl[])
            n104 = Array Subset(array=w266, index=192, length=w278) -> (w270:sgl[])
            n105 = Array Subset(array=w266, index=384, length=w278) -> (w274:sgl[])
            n106 = Array Subset(array=w266, index=576, length=w278) -> (w272:sgl[])
            n107 = call "Convert to Dynamic Data3"("Array"=w270) -> ("Dynamic Data Type"=w269:dynamicdata)  [unwired: 3 in]
            n108 = call "Convert to Dynamic Data"("Array"=w274) -> ("Dynamic Data Type"=w273:dynamicdata)  [unwired: 3 in]
            n109 = call "Convert to Dynamic Data4"("Array"=w268) -> ("Dynamic Data Type"=w267:dynamicdata)  [unwired: 3 in]
            n110 = call "Convert to Dynamic Data2"("Array"=w272) -> ("Dynamic Data Type"=w271:dynamicdata)  [unwired: 3 in]
            n111 = Merge Signals(w267, w269, w273, w271) -> (→"Waveform Graph":dynamicdata)
          }
        }
        "Modbus_Master-Error" <- w177
        n112 = Unbundle By Name(w177) -> ("status"=w197:bool)
        n113 = Boolean To (0,1)(Boolean=w197) -> (0, 1=w194:i16)
        n114 = feedback #1() -> (w195:i16)  [unwired: 1 in]
        "RX/TX_Errors" <- w195
        n115 = Add(x=w195, y=w194) -> (x+y=w196:i16)
        n116 = feedback-in #1(w196) -> ()
      }
      n117 = call-dynamic "Close.vi"("error in (no error)"=w6, "Modbus master in"=w5) -> ()  [unwired: 9 in, 1 out]
    }
  }
